vi "Main.vi"(11 "Module Admin":refnum<class "Delacor_lib_QMH_Module Admin.lvclass">) -> ()   [LabVIEW 2020, in "Panther Dashboard.lvlib"]
doc: "Panther Dashboard For DQMH®\n\nDeveloped and maintained by:\nPantherLAB\n\nDeveloper:\n\n» Enrique Noé Arias"
uses:
  Panther Dashboard.lvlib
  <vilib>/Delacor/Delacor QMH/Libraries/Module Admin_class/Delacor_lib_QMH_Module Admin.lvclass
  Controls/Add Event.ctl
  Controls/Remove Event.ctl
  Controls/Convert Event.ctl
  Controls/Rename event.ctl
  Controls/Info.ctl
  Controls/Add New Module.ctl
  Controls/Rename Module.ctl
  Controls/Validate Module.ctl
  Controls/Template.ctl
  Controls/Unit Test.ctl
  Controls/Create Real Time API.ctl
  Controls/Antidoc Open.ctl
  Controls/Antidoc Create.ctl
  Controls/DQMH Help.ctl
  Controls/Add Helper Loop.ctl
  Controls/home.ctl
  Controls/Duplicate Event.ctl
  Controls/Duplicate Module.ctl
  Controls/Configuration.ctl
  Controls/Call HSE-Ify.ctl
  Module Data--cluster.ctl
  Class/Project/Project.lvclass
  C:/GitClones/PantherDashboard/src/LabVIEW/Panther Dashboard/Class/LabVIEWItem/LabVIEWItem.lvclass
  Class/Library/Library.lvclass
  Class/VI/VI.lvclass
  Class/LabVIEWItem/Item Type--enum.ctl
  Module type--enum.ctl
  DQMH Tools Menu--enum.ctl
  Launch DQMH Scripting Tools Argument--cluster.ctl
  <vilib>/Delacor/Delacor QMH/Libraries/Message Queue_class/Delacor_lib_QMH_Message Queue.lvclass/Delacor_lib_QMH_Message Queue.ctl
  Execute Default Event Request Argument--cluster.ctl
  Tree DQMH Selection Argument--cluster.ctl
  Scan DQMH Modules Argument--cluster.ctl
  Stop Argument--cluster.ctl
  Generate Project Documentation Argument--cluster.ctl
  Show About Argument--cluster.ctl
  Update Module ID Argument--cluster.ctl
  Save Library Description Argument--cluster.ctl
  Save VI Description Argument--cluster.ctl
  Open Documentation Argument--cluster.ctl
  Save Project Documentation Argument--cluster.ctl
  Load Project From Path Argument--cluster.ctl
  Add DQMH Module to Current Scan Argument--cluster.ctl
  Highlight Item Argument--cluster.ctl
  Add new Module by Path Argument--cluster.ctl
  Refresh Module By Name Argument--cluster.ctl
  Remove Module By Name Argument--cluster.ctl
  <vilib>/Delacor/Delacor QMH/Libraries/Module Admin_class/Delacor_lib_QMH_Module Admin.lvclass/Delacor_lib_QMH_Module Admin.ctl
  Class/Project/Project.lvclass/Project.ctl
  Public VIs names--enum.ctl
  Class/LabVIEWItem/LabVIEWItem.lvclass/LabVIEWItem.ctl
  Documentation--cluster.ctl
  Class/Library/Library.lvclass/Library.ctl
  <vilib>/Delacor/Delacor QMH/Libraries/Message Queue_class/Delacor_lib_QMH_Enqueue Message (Single).vi
  <vilib>/Delacor/Delacor QMH/Libraries/Module Admin_class/Delacor_lib_QMH_Get External Launch.vi
  Class/LabVIEWItem/Read Item Name.vi
  Class/LabVIEWItem/Read Item Path.vi
  Class/LabVIEWItem/Read Item Type.vi
  Class/Project/Read Project Ref.vi
  Class/LabVIEWItem/Read Item Description.vi
  Class/Library/Read Type.vi
  Class/LabVIEWItem/Write Item Description.vi
  Panther Dashboard--global.vi
  <vilib>/Platform/browser.llb/Open URL in Default Browser (path).vi
  <vilib>/Utility/error.llb/Error Cluster From Error Code.vi
  <vilib>/ErrorRing/Error Ring.xnode
  <vilib>/Delacor/Delacor QMH/Libraries/Message Queue_class/Delacor_lib_QMH_Message Queue.lvclass
  <vilib>/Delacor/Delacor QMH/Libraries/Scripting API/DQMH_Scripting API.lvlib
  ContextHelp/ContextHelp.lvlib
  Class/LabVIEWItem/LabVIEWItem.lvclass
panel:
  in  "Context Help Panther":T1 caption="Doc Editor"
  in  "Duplicate Event":T2
  in  "Add Event":T3
  in  "Remove Event":T4 caption="Remove"
  in  "Convert Event":T5 caption="Convert"
  in  "Rename Event":T6 caption="Rename"
  in  "HSE-Ifi Module":T7
  in  "Duplicate Module":T8
  in  "Add Helper Loop to Module":T9
  in  "Add New Module":T10 caption="Add"
  in  "Rename Module":T11 caption="Rename"
  in  "Validate Module":T12 caption="Validate"
  in  "Create Module Template":T13 caption="Template"
  in  "Add Unit Test Module":T14 caption="Unit Test"
  in  "Create RT Tester Module":T15 caption="RT Tester"
  in  "Open Antidoc Output":T16 caption="Open"
  in  "Generate Antidoc":T17 caption="Antidoc"
  in  "Config":T18
  in  "About Panther":T19 caption="About"
  in  "Home":T20
  in  "Modules Tree":string(tree)
  in  "Module ID":i32=-1 min=-1 max=1000 step=1 format="Module ID %d"
  out "String Control":string
  out "error out":errorcluster
  out "Progress":i16(slide) scale=-1.0..11.0
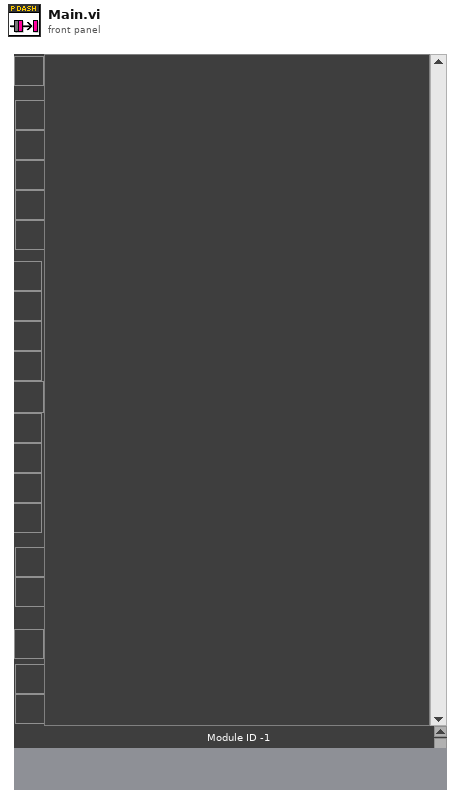
[diagram p1: front panel]
types:
  T1 = typedef "DQMH Help.ctl" = bool
  T2 = typedef "Duplicate Event.ctl" = bool
  T3 = typedef "Add Event.ctl" = bool
  T4 = typedef "Remove Event.ctl" = bool
  T5 = typedef "Convert Event.ctl" = bool
  T6 = typedef "Rename event.ctl" = bool
  T7 = typedef "Call HSE-Ify.ctl" = bool
  T8 = typedef "Duplicate Module.ctl" = bool
  T9 = typedef "Add Helper Loop.ctl" = bool
  T10 = typedef "Add New Module.ctl" = bool
  T11 = typedef "Rename Module.ctl" = bool
  T12 = typedef "Validate Module.ctl" = bool
  T13 = typedef "Template.ctl" = bool
  T14 = typedef "Unit Test.ctl" = bool
  T15 = typedef "Create Real Time API.ctl" = bool
  T16 = typedef "Antidoc Open.ctl" = bool
  T17 = typedef "Antidoc Create.ctl" = bool
  T18 = typedef "Configuration.ctl" = bool
  T19 = typedef "Info.ctl" = bool
  T20 = typedef "home.ctl" = bool
  T21 = typedef "Panther Dashboard.lvlib/Broadcast Events--cluster.ctl" = cluster{"Module Did Init":refnum<user-event>, "Status Updated":refnum<user-event>, "Error Reported":refnum<user-event>, "Module Did Stop":refnum<user-event>, "Update Module Execution Status":refnum<user-event>, "References Updated":refnum<user-event>, "Progress updated":refnum<user-event>, "Scale Updated":refnum<user-event>, "Connector Pane Updated":refnum<user-event>, "Documentation Updated":refnum<user-event>, "Module Type Updated":refnum<user-event>, "Project Description Updated":refnum<user-event>}
  T22 = typedef "Panther Dashboard.lvlib/Request Events--cluster.ctl" = cluster{"Stop Module":refnum<user-event>, "Show Panel":refnum<user-event>, "Hide Panel":refnum<user-event>, "Get Module Execution Status":refnum<user-event>, "Show Diagram":refnum<user-event>, "Scan DQMH Modules":refnum<user-event>, "Tree DQMH Selection":refnum<user-event>, "Open Module API Tester":refnum<user-event>, "Execute Default Event Request":refnum<user-event>, "Launch DQMH Scripting Tools":refnum<user-event>, "Generate Project Documentation":refnum<user-event>, "Show About":refnum<user-event>, "Update Module ID":refnum<user-event>, "Save Library Description":refnum<user-event>, "Save VI Description":refnum<user-event>, "Open Documentation":refnum<user-event>, "Save Project Documentation":refnum<user-event>, "Register controls Mouse Enter":refnum<user-event>, "Load Project From Path":refnum<user-event>, "Add DQMH Module to Current Scan":refnum<user-event>, "Highlight Item":refnum<user-event>, "Update Status":refnum<user-event>, "Add new Module by Path":refnum<user-event>, "Refresh Module By Name":refnum<user-event>, "Remove Module By Name":refnum<user-event>}
  T23 = typedef "ContextHelp.lvlib/Broadcast Events--cluster.ctl" = cluster{"Module Did Init":refnum<user-event>, "Status Updated":refnum<user-event>, "Error Reported":refnum<user-event>, "Module Did Stop":refnum<user-event>, "Update Module Execution Status":refnum<user-event>}
  T24 = typedef "Panther Dashboard.lvlib/LabVIEWItem.lvclass/Item Type--enum.ctl" = enum16{"Requests", "Broadcasts", "Request and Wait for Reply", "Round Trip", "» Public API VIs", "» Constant VIs", "» Error VIs", "Module", "Project", "No Drag Selection"}
  T25 = typedef "Panther Dashboard.lvlib/Module Data--cluster.ctl" = cluster{"Project":refnum<class "Project.lvclass">, "Current Selection":cluster{"Library":refnum<class "Library.lvclass">, "VI":refnum<class "VI.lvclass">}, "Module ID":i32, "Tree Selection":string}
  T26 = typedef "Panther Dashboard.lvlib/Module type--enum.ctl" = enum16{"Singleton", "Cloneable"}
  T27 = typedef "Panther Dashboard.lvlib/Launch DQMH Scripting Tools Argument--cluster.ctl" = cluster{"Scripting Tool":T28}
  T28 = typedef "Panther Dashboard.lvlib/DQMH Tools Menu--enum.ctl" = enum16{"Create New DQMH Event", "Remove DQMH Event", "Convert DQMH Event", "Rename DQMH Event", "Add New DQMH Module", "Create RT Tester", "Rename DQMH Module", "Validate DQMH Module", "Create DQMH Module Template", "New DQMH  Unit Test", "Add Helper Loop to DQMH Module", "Duplicate Event", "HSE-ify DQMH Module", "Duplicate Module"}
  T29 = typedef "Panther Dashboard.lvlib/Execute Default Event Request Argument--cluster.ctl" = cluster{"Event Name":string}
  T30 = typedef "Panther Dashboard.lvlib/Tree DQMH Selection Argument--cluster.ctl" = cluster{"Tree Sel":string}
  T31 = typedef "Panther Dashboard.lvlib/Scan DQMH Modules Argument--cluster.ctl" = cluster{"Include Dependencies":bool, "Scan All":bool, "Project":string, "Target":string}
  T32 = enum32{"invalid lock state", "Not Locked", "Locked (No Password)", "Password-protected"}
  T33 = typedef "Panther Dashboard.lvlib/Stop Argument--cluster.ctl" = cluster{"Origin":string, "Exit via Stop Module Req?":bool, "Wait for Module to stop?":bool}
  T34 = typedef "Panther Dashboard.lvlib/Generate Project Documentation Argument--cluster.ctl" = cluster{"Boolean":bool}
  T35 = typedef "Panther Dashboard.lvlib/Show About Argument--cluster.ctl" = cluster{"Boolean":bool}
  T36 = typedef "Panther Dashboard.lvlib/Update Module ID Argument--cluster.ctl" = cluster{"New ID":i32}
  T37 = typedef "Panther Dashboard.lvlib/Save Library Description Argument--cluster.ctl" = cluster{"Library Description":string}
  T38 = typedef "Panther Dashboard.lvlib/Save VI Description Argument--cluster.ctl" = cluster{"VI Description":string}
  T39 = typedef "Panther Dashboard.lvlib/Open Documentation Argument--cluster.ctl" = cluster{"Boolean":bool}
  T40 = typedef "Panther Dashboard.lvlib/Save Project Documentation Argument--cluster.ctl" = cluster{"Project Description":string}
  T41 = typedef "Panther Dashboard.lvlib/Load Project From Path Argument--cluster.ctl" = cluster{"Project Path":path}
  T42 = typedef "Panther Dashboard.lvlib/Add DQMH Module to Current Scan Argument--cluster.ctl" = cluster{"Include Dependencies":bool}
  T43 = typedef "Panther Dashboard.lvlib/Highlight Item Argument--cluster.ctl" = cluster{"Item Tag":string}
  T44 = typedef "Panther Dashboard.lvlib/Add new Module by Path Argument--cluster.ctl" = cluster{"Module Folder":path, "Module Name":string}
  T45 = typedef "Panther Dashboard.lvlib/Refresh Module By Name Argument--cluster.ctl" = cluster{"Module Name":string}
  T46 = typedef "Panther Dashboard.lvlib/Remove Module By Name Argument--cluster.ctl" = cluster{"Module Name":string}
  T47 = typedef "Panther Dashboard.lvlib/Public VIs names--enum.ctl" = enum16{"Start Module.vi", "Synchronize Module Events.vi", "Obtain Broadcast Events for Registration.vi", "Null Broadcast Events--constant.vi", "Stop Module.vi", "Load Module.vi", "Obtain Default Broadcast Events.vi"}
  T48 = typedef "Panther Dashboard.lvlib/Documentation--cluster.ctl" = cluster{"Module Description":string, "Event Description":string}
  T49 = typedef "Panther Dashboard.lvlib/Pdash Style--cluster.ctl" = cluster{"Gris Obscuro Azul":u32, "Gris Medio Azul":u32, "Gris Claro Azul":u32, "Amarillo":u32, "Text color":u32, "Transparent":u32, "Fuente":string, "Text.Font:Size":u32}
  T50 = cluster{"Library":refnum<class "Library.lvclass">, "VI":refnum<class "VI.lvclass">}
  T51 = typedef "Panther Dashboard.lvlib/Helper Loop--cluster.ctl" = cluster{"Main.vi Refs":refnum<vi>[], "Libraries Names":string[], "Modules Types":T26[], "Dependencies":bool[], "Project Name":string, "HSE Module":bool[], "Glyphs Map":map{T52, i32}, "TreeControl Ref":refnum<vi>}
  T52 = typedef "Panther Dashboard.lvlib/Glyphs--enum.ctl" = enum16{"Singleton", "SingletonRun", "SingletonDepencencies", "SingletonDependenciesRun", "Cloneable", "CloneableRun", "CloneableDependencies", "CloneableDependenciesRun", "HSE_Singleton", "HSE_SingletonRun", "HSE_SingletonDependencies", "HSE_SingletonDependenciesRun", "HSE_Cloneable", "HSE_CloneableRun", "HSE_CloneableDependencies", "HSE_CloneableDependenciesRun", "DQMH_Proj", "HSE_Proj", "Bad"}
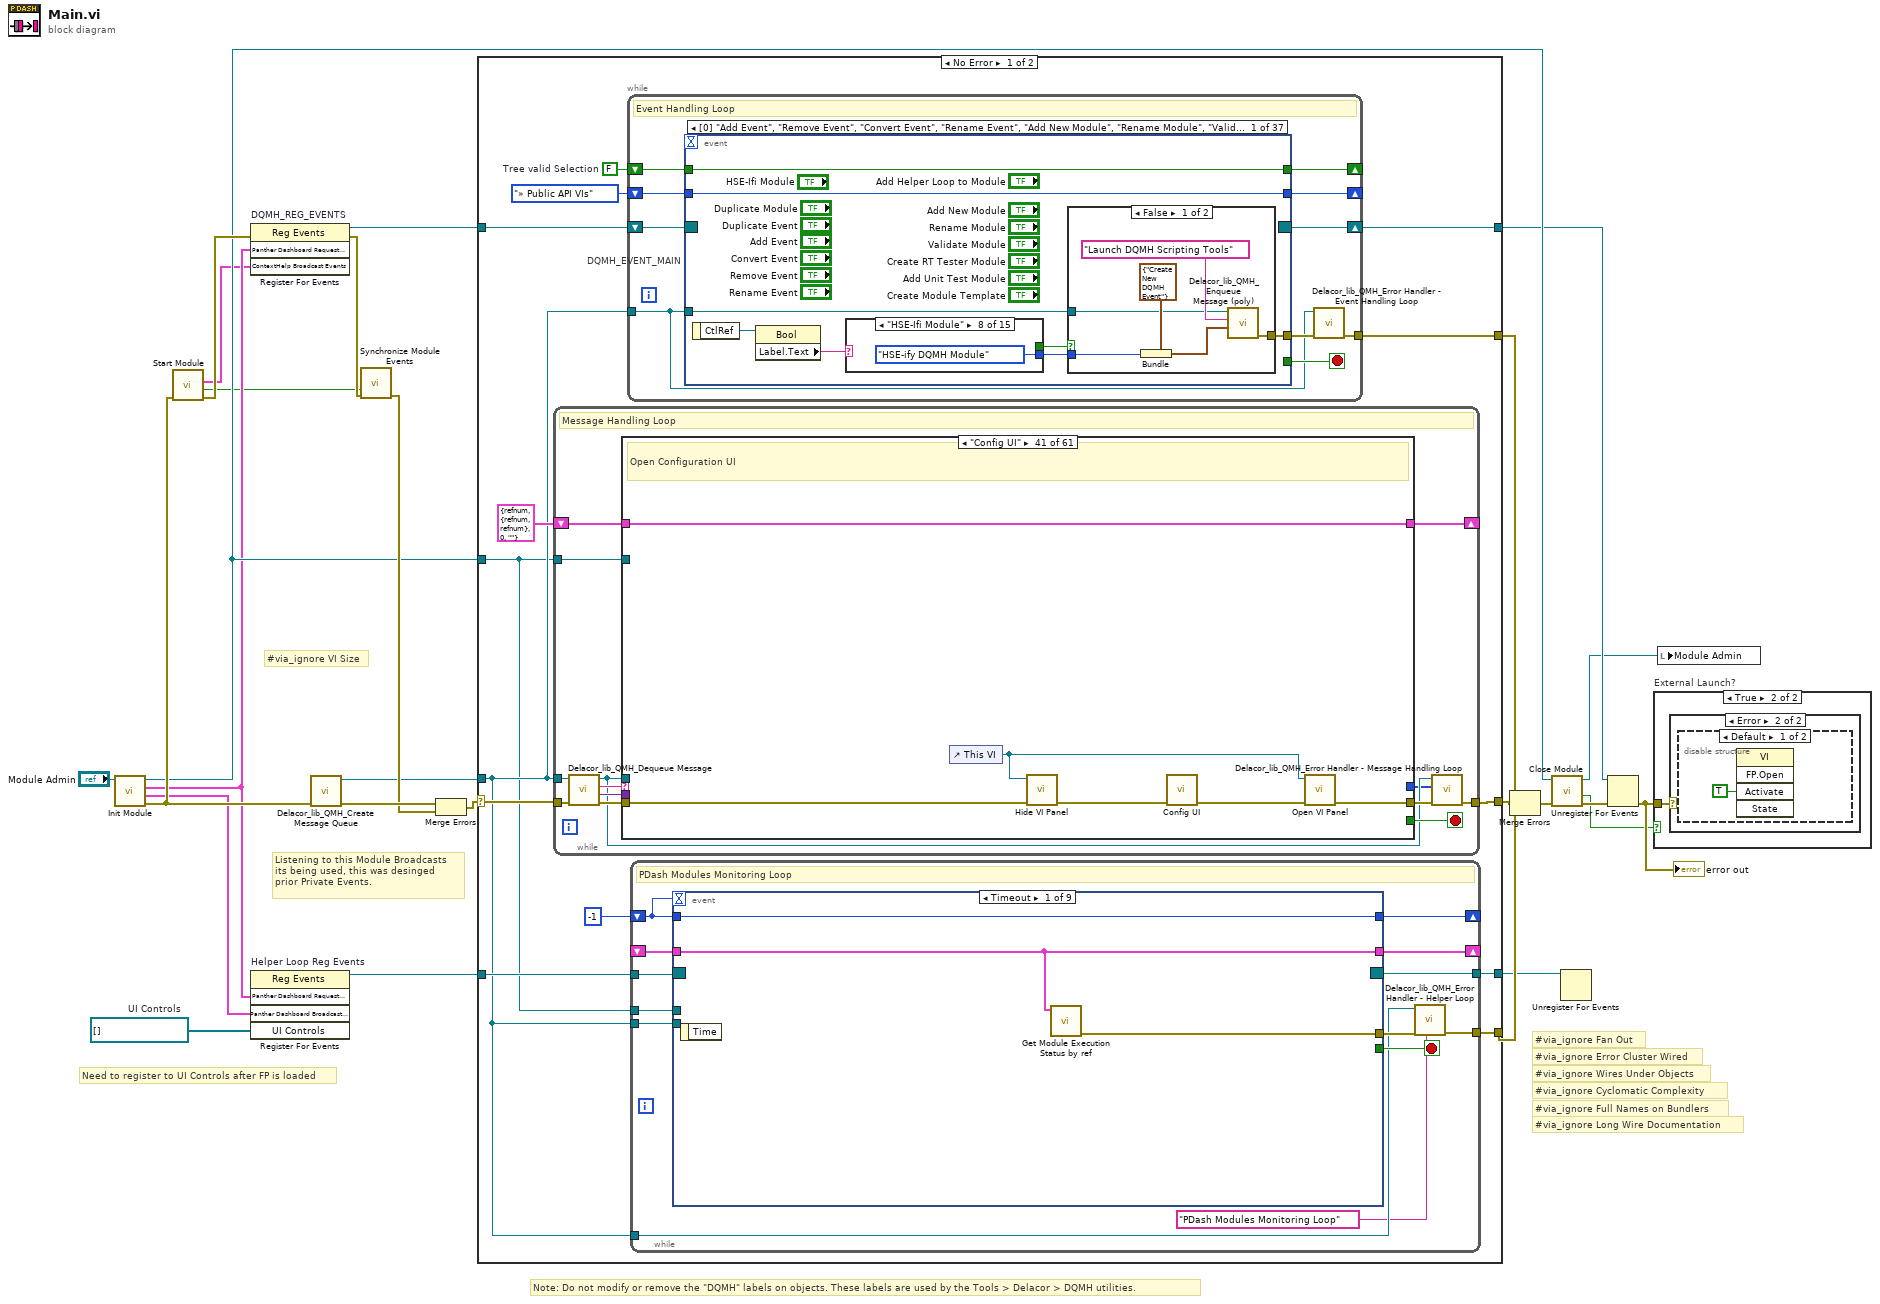
[diagram p0: block diagram]
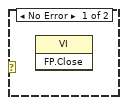
[diagram p3: hidden frame]
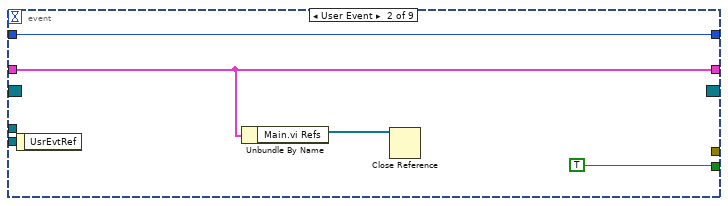
[diagram p5: hidden frame]
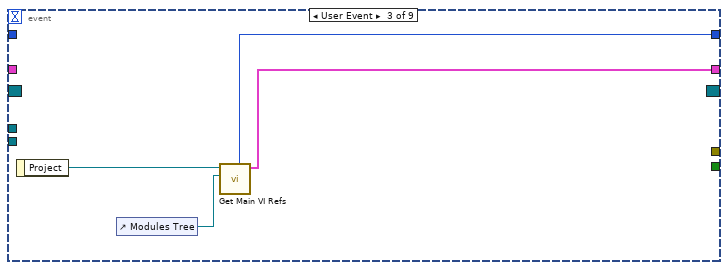
[diagram p6: hidden frame]
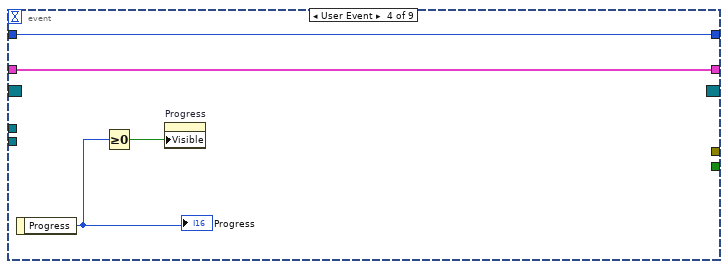
[diagram p7: hidden frame]
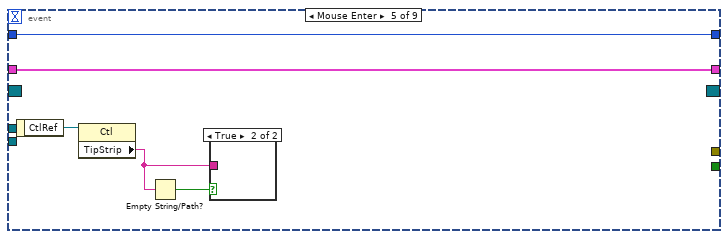
[diagram p8: hidden frame]
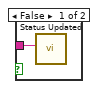
[diagram p9: hidden frame]
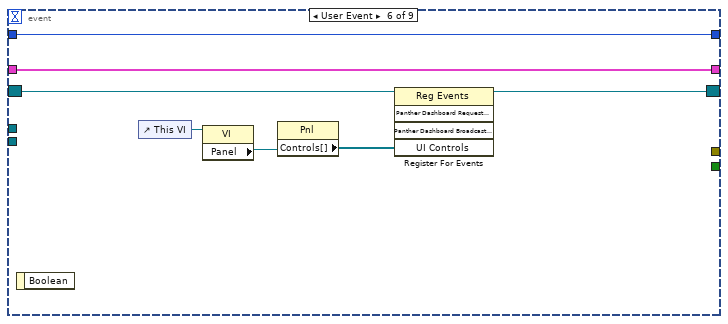
[diagram p10: hidden frame]
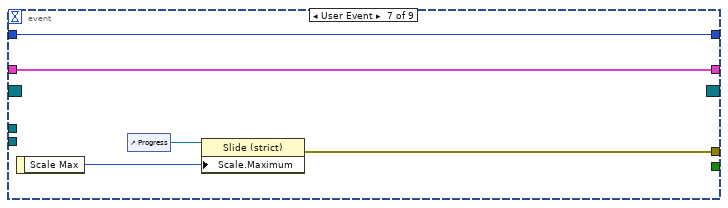
[diagram p11: hidden frame]
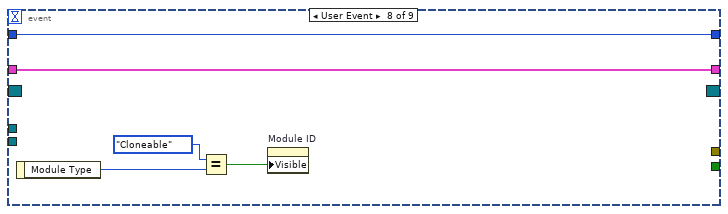
[diagram p12: hidden frame]
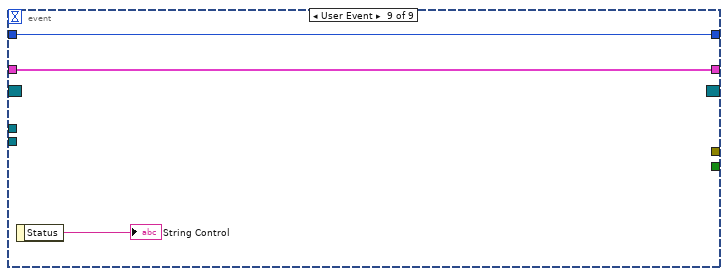
[diagram p13: hidden frame]
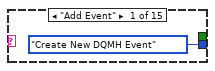
[diagram p15: hidden frame]
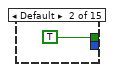
[diagram p16: hidden frame]
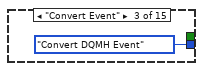
[diagram p17: hidden frame]
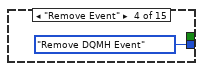
[diagram p18: hidden frame]
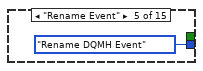
[diagram p19: hidden frame]
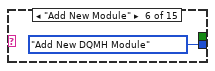
[diagram p20: hidden frame]
diagram:
  w1 = refnum<vi>[] []  # UI Controls
  # "Listening to this Module Broadcasts\nits being used, this was desinged\nprior Private Events."
  # "#via_ignore Long Wire Documentation"
  # "#via_ignore Full Names on Bundlers"
  # "Need to register to UI Controls after FP is loaded"
  # "#via_ignore VI Size"
  # "#via_ignore Fan Out"
  # "#via_ignore Cyclomatic Complexity"
  # "#via_ignore Wires Under Objects"
  # "#via_ignore Error Cluster Wired"
  # "Note: Do not modify or remove the \"DQMH\" labels on objects. These labels are used by the Tools > Delacor > DQMH utilities."
  n1 = call "Init Module.vi"("Singleton Module Admin in"="Module Admin") -> ("error out"=w15:errorcluster, "Panther Dashboard Broadcast Events"=w4:T21, "Panther Dashboard Request Events"=w5:T22, "Singleton Module Admin out"=w14:refnum<class "Delacor_lib_QMH_Module Admin.lvclass">)  [unwired: 7 in]
  n2 = call "Start Module.vi"("error in"=w15) -> ("error out"=w17:errorcluster, "Wait for Event Sync?"=w3:bool, "ContextHelp Broadcast Events"=w2:T23)  [unwired: 6 in, 2 out]
  n3 = register-events "DQMH_REG_EVENTS"(error in=w17, w5, w2) -> (reference out=w12:refnum<event-registration>, error out=w18:errorcluster)  [unwired: 1 in]
  n4 = register-events "Helper Loop Reg Events"(w5, w4, w1) -> (reference out=w7:refnum<event-registration>)  [unwired: 2 in, 1 out]
  n5 = call <vilib>:"Delacor_lib_QMH_Create Message Queue.vi"("error in"=w15) -> ("error out"=w21:errorcluster, "Message Queue"=w11:refnum<class "Delacor_lib_QMH_Message Queue.lvclass">)  [unwired: 9 in]
  n6 = call "Synchronize Module Events.vi"("error in"=w18, "Wait for Event Sync?"=w3) -> ("error out"=w16:errorcluster)  [unwired: 9 in]
  n7 = Merge Errors(w21, w16) -> (w20:errorcluster)
  n8 = case shown="No Error" w20 {
    selector: w20 -> [w38 w1095]
    tunnel: [w40 w1094] -> w26
    tunnel: [w36 w1093] -> w13
    tunnel: w12 -> [w34 w1093]
    tunnel: w11 -> [w29 w1089]
    tunnel: [w39 _] -> w24
    tunnel: w14 -> [w28 w1090]
    tunnel: w7 -> [w33 w1088]
    tunnel: [w32 w1088] -> w6
    tunnel: [w37 _] -> w19
    frame No Error {
      w30 = FALSE  # Tree valid Selection
      n9 = while {
        tunnel: w29 -> [w456]
        shift-right: [w460] -> _
        shift-left: T25 {"Project"=refnum, "Current Selection"={"Library"=refnum, "VI"=refnum}, "Module ID"=0, "Tree Selection"=""} ("Data Cluster") -> [w461]
        tunnel: w38 -> [w464]
        tunnel: [w462] -> w40
        tunnel: w28 -> [w454]
        stop <- w459 stop-if-true
        # "Message Handling Loop"
        n10 = call-dynamic "Delacor_lib_QMH_Dequeue Message.vi"("error in"=w464, "Message Queue in"=w456) -> ("error out"=w463:errorcluster, "Message Data"=w457:variant, "Message"=w458:string, "Message Queue out"=w455:refnum<class "Delacor_lib_QMH_Message Queue.lvclass">)  [unwired: 6 in]
        n11 = case "DQMH_MESSAGE_CASES" shown="\"Config UI\"" w458 {
          selector: w458 -> [_ _ _ _ _ _ _ _ _ _ _ _ _ _ _ _ _ _ _ _ _ _ _ _ _ _ _ _ _ _ _ _ _ _ _ _ _ _ _ _ _ _ _ _ _ _ _ _ _ _ _ _ _ _ _ _ _ w1037 _ _ _]
          tunnel: w455 -> [_ _ _ _ _ _ _ _ _ _ _ _ _ _ _ _ w606 w629 _ _ _ _ _ _ _ _ _ _ _ _ _ _ _ _ _ _ _ _ _ _ _ _ _ _ w871 _ _ _ _ _ _ _ _ _ _ w1002 w1029 _ _ _ _]
          tunnel: w463 -> [w485 w488 w494 w501 w507 w515 w526 w540 w545 w548 w561 w570 w575 w581 w586 w594 w608 w631 w648 w654 w663 w668 w670 w678 w680 w689 w694 w707 w726 w754 _ w766 w774 w777 w794 w809 w814 w819 w821 w830 w836 w844 w866 w868 w882 w892 w898 w909 w912 w921 w931 w951 w974 w988 w999 w1009 w1035 w1039 w1059 w1076 w1086]
          tunnel: [w483 w488 w495 w502 w509 w514 w525 w538 w544 w549 w558 w568 w573 w579 w587 w595 w607 w630 w647 w653 w662 w667 w670 w675 w680 w685 w693 w705 w724 w755 w763 w767 w772 w787 w793 w803 w813 w818 w821 w826 w833 w843 w865 w868 w881 w891 w896 w910 w912 w919 w928 w949 w970 w986 w999 w1005 w1032 w1040 w1057 w1074 w1085] -> w465
          tunnel: w461 -> [w475 w487 w492 w499 w506 w513 w517 w531 w542 w547 w557 w567 w572 w578 w585 w593 w602 w624 w646 w652 w661 w666 w669 w674 w679 w684 w692 w700 w723 w752 w760 w765 w771 w783 w792 w802 w812 w817 w820 w825 w832 w842 w858 w867 w875 w890 w895 w905 w911 w915 w924 w943 w962 w981 w998 w1004 w1019 w1038 w1053 w1069 w1080]
          tunnel: [w481 w487 w492 w499 w506 w513 w520 w528 w541 w546 w556 w567 w572 w578 w585 w593 w600 w623 w646 w652 w661 w666 w669 w674 w679 w684 w692 w700 w723 w752 w760 w765 w771 w783 w790 w802 w812 w817 w820 w825 w832 w838 w850 w867 w874 w890 w895 w905 w911 w915 w922 w942 w962 w980 w998 w1004 w1019 w1038 w1052 w1068 w1079] -> w460
          tunnel: [_ _ _ _ _ _ _ _ _ _ _ _ _ _ _ _ _ _ _ _ _ _ _ _ _ _ _ _ _ _ _ _ _ _ _ _ _ _ _ _ _ _ _ _ _ _ _ _ _ _ _ _ _ _ _ _ w1028 _ _ _ _] -> w459
          tunnel: w457 -> [_ _ _ _ _ _ w522 w537 _ _ _ w566 _ _ _ _ _ _ _ _ _ _ _ _ _ _ _ w703 _ _ _ _ _ _ w791 _ _ _ _ w824 _ w841 w861 _ w878 _ _ _ _ w917 w927 w947 w969 w985 _ w1003 w1027 _ w1056 w1073 w1083]
          tunnel: w454 -> [w482 _ _ _ _ _ _ _ _ _ _ _ _ _ _ _ _ _ _ _ _ _ _ _ _ _ _ _ _ _ _ _ _ _ _ _ _ _ _ _ _ _ _ _ _ _ _ _ _ _ _ _ _ _ _ w1001 w1022 _ _ _ _]
          tunnel: [_ _ _ _ _ _ _ _ _ _ _ _ _ _ _ _ _ _ _ _ _ _ _ _ _ _ _ _ i32[] [5000, 1026, 43] ("specific error code to clear (0: all)") _ _ _ _ _ _ _ _ _ _ _ _ _ _ _ _ _ _ _ _ _ _ _ _ _ _ _ _ _ _ _ _] -> w453
          frame "Initialize" {
            # "Initialize - Any operation that needs to be done before the module can receive messages. Synchronize Caller Events.vi will inform Start Module.vi that the module has launched and is ready to receive messages. Module Did Init.vi will broadcast that the module initialized."
            n12 = call "Synchronize Caller Events.vi"("error in (no error)"=w485, "Singleton Module Admin in"=w482) -> ("error out"=w484:errorcluster, "Singleton Module Admin out"=w474:refnum<class "Delacor_lib_QMH_Module Admin.lvclass">)  [unwired: 8 in]
            n13 = property on="Modules Tree" class="Tree (strict)"("Allow Item Drag"=TRUE ("Drag/Drop:Allow Dragging"), "SelColor"=u32 5987163) -> ()  [unwired: 2 in, 2 out]
            n14 = call "Module Name--constant.vi"() -> ("Module Name"=w479:string)  [unwired: 11 in]
            n15 = call "Module Did Init.vi"("error in (no error)"=w484, "Initialized?"=TRUE, "Origin"=w479) -> ("error out"=w483:errorcluster)  [unwired: 8 in]
            n16 = property class="Module Admin"(reference=w474) -> ("Accessors:External Launch"=w473:bool)  [unwired: 1 in, 2 out]
            n17 = case shown="False" w473 {
              frame False {
                n18 = call "Show Panel.vi"() -> ()  [unwired: 11 in, 1 out]
              }
              frame True {
              }
            }
            n19 = call "Get Panther Dashboard Version.vi"() -> ("Panther Dashboard Version"=w470:string)  [unwired: 11 in]
            n20 = Format Into String(format string="Panther Dashboard for DQMH %s" ("String"), w470) -> (resulting string=w469:string)  [unwired: 2 in, 1 out]
            n21 = control-ref of="This VI"() -> (w472:refnum<vi>)
            n22 = flat-sequence {
              tunnel: [w486] -> w468
              frame #0 {
                n23 = call "PDash Branding.vi"() -> ()  [unwired: 12 in]
                n24 = call "Pdash Style--constant.vi"() -> ("Style"=w486:T49)  [unwired: 11 in]
              }
            }
            n25 = property class="VI"(reference=w472, "Front Panel.Title"=w469) -> ()  [unwired: 1 in, 2 out]
            n26 = Unbundle By Name(w468) -> ("Gris Medio Azul"=w467:u32)
            n27 = call "Status Updated.vi"("Status"=w469) -> ()  [unwired: 10 in, 1 out]
            n28 = control-ref of="Pane Bottom"() -> (w466:refnum<vi>)
            n29 = Bundle By Name(cluster=w475, "Module ID"=-1) -> (w481:T25)
            n30 = property class="Pane"(reference=w466, "PaneColor"=w467) -> ()  [unwired: 1 in, 2 out]
          }
          frame "--------MODULE-----------" {
          }
          frame "Module Data--cluster.ctl" {
            # "Open Module's Data Typedef"
            n31 = Unbundle By Name(w492) -> ("Project"=w490:refnum<class "Project.lvclass">, "Current Selection.Library"=w491:refnum<class "Library.lvclass">)
            n32 = call "Read Main App Inst Ref.vi"("error in (no error)"=w494, "Project in"=w490) -> ("error out"=w493:errorcluster, "Main App Inst Ref"=w489:refnum<vi>)  [unwired: 7 in, 1 out]
            n33 = call "Open Module Data Typedef.vi"("App Instance"=w489, "error in"=w493, "Library in"=w491) -> ("error out"=w495:errorcluster)  [unwired: 7 in, 1 out]
          }
          frame "Main.vi Block Diagram" {
            n34 = Unbundle By Name(w499) -> ("Project"=w497:refnum<class "Project.lvclass">, "Current Selection.Library"=w498:refnum<class "Library.lvclass">)
            n35 = call "Read Main App Inst Ref.vi"("error in (no error)"=w501, "Project in"=w497) -> ("error out"=w500:errorcluster, "Main App Inst Ref"=w496:refnum<vi>)  [unwired: 7 in, 1 out]
            n36 = call "Open Module Main Block Diagram.vi"("App Instance"=w496, "error in"=w500, "Library in"=w498) -> ("error out"=w502:errorcluster)  [unwired: 7 in, 1 out]
          }
          frame "Main.vi Front Panel" {
            n37 = Unbundle By Name(w506) -> ("Project"=w504:refnum<class "Project.lvclass">, "Current Selection.Library"=w505:refnum<class "Library.lvclass">)
            n38 = call "Read Main App Inst Ref.vi"("error in (no error)"=w507, "Project in"=w504) -> ("error out"=w508:errorcluster, "Main App Inst Ref"=w503:refnum<vi>)  [unwired: 7 in, 1 out]
            n39 = call "Open Module Main Front Panel.vi"("App Instance"=w503, "error in"=w508, "Library in"=w505) -> ("error out"=w509:errorcluster)  [unwired: 7 in, 1 out]
          }
          frame "API Tester" {
            w510 = TRUE  # Run API Tester?
            # "Open the API Tester from the current DQMH Module Selected"
            n40 = Unbundle By Name(w513) -> ("Project"=w511:refnum<class "Project.lvclass">, "Current Selection.Library"=w512:refnum<class "Library.lvclass">)
            n41 = call "Open API Tester.vi"("Run API Tester?"=w510, "error in"=w515, "Library"=w512, "Project"=w511) -> ("error out"=w514:errorcluster)  [unwired: 7 in]
          }
          frame "Scan DQMH Modules" {
            # "Scan DQMH Modules in the project, builds a Project Object and draws a Tree with the scanned Project."
            n42 = Variant To Data(error in=w526, type=T31 {"Include Dependencies"=FALSE, "Scan All"=FALSE, "Project"="", "Target"=""} ("Scan DQMH Modules Argument"), Variant=w522) -> (data=w518:T31, error out=w524:errorcluster)
            n43 = call <vilib>:"Set Busy.vi"("error in (no error)"=w524) -> ()  [unwired: 9 in, 2 out]
            n44 = control-ref of="Modules Tree"() -> (w519:refnum<vi>)
            n45 = call "Scan DQMH Modules from Project.vi"("TreeControl in"=w519, "Data Cluster In"=w517, "error in"=w524, "Scan DQMH Modules Argument"=w518) -> ("error out"=w523:errorcluster, "Data Cluster Out"=w520:T25)  [unwired: 6 in]
            n46 = call <vilib>:"Unset Busy.vi"("error in (no error)"=w523) -> ()  [unwired: 10 in, 1 out]
            n47 = call "Progress updated.vi"("error in"=w523, "Progress"=i16 -1) -> ()  [unwired: 9 in, 1 out]
            n48 = call "Show Panel.vi"("error in (no error)"=w523) -> ("error out"=w525:errorcluster)  [unwired: 10 in]
          }
          frame "Launch DQMH Scripting Tools" {
            # "Launch the DQMH Scripting Tools"
            n49 = Variant To Data(error in=w540, type=T27 {"Scripting Tool"=enum."Create New DQMH Event"} ("Launch DQMH Scripting Tools Argument"), Variant=w537) -> (data=w535:T27, error out=w539:errorcluster)
            n50 = Unbundle By Name(w535) -> ("Scripting Tool"=w532:T28)
            n51 = Format Into String(format string="Executing DQMH: %s", w532) -> (resulting string=w534:string)  [unwired: 2 in, 1 out]
            n52 = call "Status Updated.vi"("Status"=w534) -> ()  [unwired: 10 in, 1 out]
            n53 = Unbundle By Name(w531) -> ("Project"=w530:refnum<class "Project.lvclass">, "Current Selection"=w529:T50)
            n54 = call "Launch DQMH Tools by menu.vi"("error in"=w539, "DQMH Tools"=w532, "Current Selection In"=w529, "Project In"=w530) -> ("error out"=w538:errorcluster, "Project Out"=w527:refnum<class "Project.lvclass">)  [unwired: 6 in]
            n55 = Bundle By Name(cluster=w531, "Project"=w527) -> (w528:T25)
          }
          frame "(X) Exclude Module from Scan" {
            # "To Exclude a Module form the current Scan, this is specially usefull when dealing with dependencies that were removed from the project."
            n56 = control-ref of="Modules Tree"() -> (w543:refnum<vi>)
            n57 = call "Remove Module from Project.vi"("TreeControl in"=w543, "error in"=w545, "Data Cluster In"=w542) -> ("error out"=w544:errorcluster, "Data Cluster Out"=w541:T25)  [unwired: 7 in]
          }
          frame "Scan Project for Manually Added Modules" {
            # "Scan Project for Manually Added Modules"
            n58 = in-place {
              in-place-border: [w554] -> w549
              in-place-border: w548 -> [w553]
              n59 = in-place-cluster #1(w547) -> ("Project"=w551:refnum<class "Project.lvclass">)
              n60 = control-ref of="Modules Tree"() -> (w552:refnum<vi>)
              n61 = call "Add Module To Project.vi"("TreeControl in"=w552, "error in"=w553, "Project"=w551) -> ("error out"=w554:errorcluster, "Project Out"=w550:refnum<class "Project.lvclass">)  [unwired: 7 in]
              n62 = in-place-cluster #1("Project"=w550) -> (w546:T25)
            }
          }
          frame "Refresh Module" {
            # "User right click a module and selected Refresh module, this will rescan the Library for events, will redraw the tree with the current module state.\nUse this functionality when working with DQMH and Panther Dashboard wasn't running, this will put the scan up to date"
            n63 = control-ref of="Modules Tree"() -> (w555:refnum<vi>)
            n64 = call <vilib>:"Set Busy.vi"("error in (no error)"=w561) -> ("error out"=w560:errorcluster)  [unwired: 9 in, 1 out]
            n65 = call "Refresh Module.vi"("TreeControl in"=w555, "Data Cluster In"=w557, "error in"=w560) -> ("error out"=w559:errorcluster, "Data Cluster Out"=w556:T25)  [unwired: 7 in]
            n66 = call <vilib>:"Unset Busy.vi"("error in (no error)"=w559) -> ("error out"=w558:errorcluster)  [unwired: 10 in]
          }
          frame "Highlight Item" {
            # "Highligh item in Tree"
            n67 = Variant To Data(error in=w570, type=T43 {"Item Tag"=""} ("Highlight Item Argument"), Variant=w566) -> (data=w564:T43, error out=w569:errorcluster)
            n68 = Unbundle By Name(w564) -> ("Item Tag"=w562:string)
            n69 = control-ref of="Modules Tree"() -> (w563:refnum<vi>)
            n70 = call "Highlight Item in Tree.vi"("error in"=w569, "Tag"=w562, "TreeControl in"=w563) -> ("error out"=w568:errorcluster)  [unwired: 8 in]
          }
          frame "Home Screen" {
            # "User clicked the Home Button."
            n71 = call "Hide Panel.vi"("error in (no error)"=w575) -> ("error out"=w574:errorcluster)  [unwired: 10 in]
            n72 = Unbundle By Name(w572) -> ("Project"=w571:refnum<class "Project.lvclass">)
            n73 = call "Init Screen.vi"("error in"=w574) -> ("error out"=w573:errorcluster)  [unwired: 10 in]
            n74 = invoke on="Modules Tree" class="Tree (strict)" method="Edit Tree Items.Delete"() -> ()  [unwired: 5 in, 5 out]
            n75 = call "Close refs.vi"("Project"=w571) -> ()  [unwired: 10 in, 1 out]
          }
          frame "Find Module in project explorer" {
            # "Open Project Explorer Window and hilite Current Module"
            n76 = Unbundle By Name(w578) -> ("Current Selection.Library"=w577:refnum<class "Library.lvclass">, "Project"=w576:refnum<class "Project.lvclass">)
            n77 = call "Find Module In Project and Open Main.vi"("error in"=w581, "Project"=w576, "Library in"=w577) -> ("error out"=w580:errorcluster)  [unwired: 8 in]
            n78 = call "Show Panel.vi"("error in (no error)"=w580) -> ("error out"=w579:errorcluster)  [unwired: 10 in]
          }
          frame "Where is this module being Launched?" {
            # "Find all the VIS calling the Start Module.vi of the selected module library"
            n79 = call <vilib>:"Set Busy.vi"("error in (no error)"=w586) -> ("error out"=w589:errorcluster)  [unwired: 9 in, 1 out]
            n80 = Unbundle By Name(w585) -> ("Project"=w584:refnum<class "Project.lvclass">, "Current Selection.Library"=w583:refnum<class "Library.lvclass">)
            n81 = call "Find API VI.vi"("error in"=w589, "Framework VI to Find"=Public_VIs_names--enum."Start Module.vi", "Library"=w583, "Project"=w584) -> ("error out"=w588:errorcluster)  [unwired: 7 in]
            n82 = call <vilib>:"Unset Busy.vi"("error in (no error)"=w588) -> ("error out"=w587:errorcluster)  [unwired: 10 in]
          }
          frame "Where is this module being Stopped?" {
            # "Find all the VIS calling the Obtain broadcast events for registration of the selected module library"
            n83 = call <vilib>:"Set Busy.vi"("error in (no error)"=w594) -> ("error out"=w597:errorcluster)  [unwired: 9 in, 1 out]
            n84 = Unbundle By Name(w593) -> ("Project"=w591:refnum<class "Project.lvclass">, "Current Selection.Library"=w590:refnum<class "Library.lvclass">)
            n85 = call "Find API VI.vi"("error in"=w597, "Framework VI to Find"=Public_VIs_names--enum."Stop Module.vi", "Library"=w590, "Project"=w591) -> ("error out"=w596:errorcluster)  [unwired: 7 in]
            n86 = call <vilib>:"Unset Busy.vi"("error in (no error)"=w596) -> ("error out"=w595:errorcluster)  [unwired: 10 in]
          }
          frame "Create Custom --error.vi" {
            # "Create an error vi for the selected library, it opens a dialog to allow developer adding Controls to the error vi to make it more flexible."
            n87 = call <vilib>:"Set Busy.vi"("error in (no error)"=w608) -> ()  [unwired: 9 in, 2 out]
            n88 = Unbundle By Name(w602) -> ("Project"=w603:refnum<class "Project.lvclass">, "Current Selection.Library"=w604:refnum<class "Library.lvclass">)
            n89 = call "Error Code Dialog.vi"("error in"=w608, "Library"=w604, "Project"=w603) -> ("error out"=w609:errorcluster, "Cancel Out"=w605:bool, "Error Name"=w599:string, "Project out"=w601:refnum<class "Project.lvclass">, "Error VI Tag"=w598:string)  [unwired: 4 in]
            n90 = case shown="False" w605 {
              tunnel: w609 -> [w618 w620]
              tunnel: [w616 w620] -> w607
              tunnel: w606 -> [w614 _]
              tunnel: w602 -> [w613 w619]
              tunnel: w601 -> [w612 _]
              tunnel: [w611 w619] -> w600
              tunnel: w599 -> [_ _]
              tunnel: w598 -> [w610 _]
              frame False {
                n91 = call-poly <vilib>:"Delacor_lib_QMH_Enqueue Message (poly).vi"("error in"=w618, "Message"="Refresh Module", "Message Queue in"=w614) -> ("error out"=w617:errorcluster)  [unwired: 7 in, 1 out]
                n92 = Bundle By Name(cluster=w613, "Project"=w612) -> (w611:T25)
                n93 = call "Highlight Item.vi"("error in"=w617, "Item Tag"=w610) -> ("error out"=w616:errorcluster)  [unwired: 9 in]
              }
              frame True {
                # "User Cancel"
              }
            }
            n94 = call <vilib>:"Unset Busy.vi"("error in (no error)"=w607) -> ()  [unwired: 10 in, 1 out]
          }
          frame "Create Custom --constant.vi" {
            # "Creates a Constant vi to the current Library selection, it opens a dialog to add controls to it, the developer can place values to the controls and those controls will be constants connected to the connector pane."
            n95 = call <vilib>:"Set Busy.vi"("error in (no error)"=w631) -> ()  [unwired: 9 in, 2 out]
            n96 = Unbundle By Name(w624) -> ("Project"=w626:refnum<class "Project.lvclass">, "Current Selection.Library"=w625:refnum<class "Library.lvclass">)
            n97 = call "Custom Constant Dialog.vi"("error in"=w631, "Library"=w625, "Project"=w626) -> ("error out"=w632:errorcluster, "Cancel Out"=w627:bool, "New Constant VI name"=w628:string, "Error VI Tag"=w622:string, "Project out"=w621:refnum<class "Project.lvclass">)  [unwired: 4 in]
            n98 = case shown="False" w627 {
              tunnel: w632 -> [w640 w643]
              tunnel: [w639 w643] -> w630
              tunnel: w629 -> [w635 _]
              tunnel: w628 -> [_ _]
              tunnel: w624 -> [w638 w642]
              tunnel: [w637 w642] -> w623
              tunnel: w622 -> [w636 _]
              tunnel: w621 -> [w634 _]
              frame False {
                n99 = call-poly <vilib>:"Delacor_lib_QMH_Enqueue Message (poly).vi"("error in"=w640, "Message"="Refresh Module", "Message Queue in"=w635) -> ("error out"=w641:errorcluster)  [unwired: 7 in, 1 out]
                n100 = Bundle By Name(cluster=w638, "Project"=w634) -> (w637:T25)
                n101 = call "Highlight Item.vi"("error in"=w641, "Item Tag"=w636) -> ("error out"=w639:errorcluster)  [unwired: 9 in]
              }
              frame True {
              }
            }
            n102 = call <vilib>:"Unset Busy.vi"("error in (no error)"=w630) -> ()  [unwired: 10 in, 1 out]
          }
          frame "Edit 'Module Name--constant.vi' value" {
            # "Sometimes we need to update or modify the 'Module Name--constant.vi' value and we need to go to this vi, open it's block diagram and change the constant value, close the vi and save it, this script does exactly that."
            n103 = Unbundle By Name(w646) -> ("Project"=w645:refnum<class "Project.lvclass">, "Current Selection.Library"=w644:refnum<class "Library.lvclass">)
            n104 = call "Script Edit Module Name.vi"("error in"=w648, "Library"=w644, "Project"=w645) -> ("error out"=w647:errorcluster)  [unwired: 8 in]
          }
          frame "Edit 'Module Timeout--constant.vi' value" {
            w649 = FALSE  # Restore to Default
            # "Sometimes we need to update or modify the 'Module Name--constant.vi' value and we need to go to this vi, open it's block diagram and change the constant value, close the vi and save it, this script does exactly that."
            n105 = Unbundle By Name(w652) -> ("Project"=w651:refnum<class "Project.lvclass">, "Current Selection.Library"=w650:refnum<class "Library.lvclass">)
            n106 = call "Script Module Timeout.vi"("Restore to Default"=w649, "error in"=w654, "Library"=w650, "Project"=w651) -> ("error out"=w653:errorcluster)  [unwired: 7 in]
          }
          frame "Restore Timeout to Default (5000ms)" {
            w660 = TRUE  # Restore to Default
            # "Restore Timeout to Default DQMH Framework value (5000ms)"
            n107 = Unbundle By Name(w661) -> ("Project"=w656:refnum<class "Project.lvclass">, "Current Selection.Library"=w655:refnum<class "Library.lvclass">)
            n108 = property class="Library"(reference=w655) -> ("Accessors:Item Name"=w658:string)  [unwired: 1 in, 2 out]
            n109 = call "Script Module Timeout.vi"("Restore to Default"=w660, "error in"=w663, "Library"=w655, "Project"=w656) -> ("error out"=w662:errorcluster)  [unwired: 7 in]
            n110 = Format Into String(format string="Module: [%s] Timeout set to Framework Default Value (5000ms)", w658) -> (resulting string=w659:string)  [unwired: 2 in, 1 out]
            n111 = call "Status Updated.vi"("error in (no error)"=w662, "Status"=w659) -> ()  [unwired: 9 in, 1 out]
          }
          frame "Open File Library on Disk" {
            # "Open current Module Library selection on the file system"
            n112 = Unbundle By Name(w666) -> ("Current Selection.Library"=w665:refnum<class "Library.lvclass">)
            n113 = property class="Library"(reference=w665) -> ("Accessors:Item Path"=w664:path)  [unwired: 1 in, 2 out]
            n114 = call "Open File on Disk.vi"("error in"=w668, "file or directory path"=w664) -> ("error out"=w667:errorcluster)  [unwired: 9 in]
          }
          frame "---------BROADCASTS---------" {
          }
          frame "Find Code registered to this module's broadcasts" {
            # "Find all the VIS calling the Obtain broadcast events for registration of the selected module library"
            n115 = call <vilib>:"Set Busy.vi"("error in (no error)"=w678) -> ("error out"=w677:errorcluster)  [unwired: 9 in, 1 out]
            n116 = Unbundle By Name(w674) -> ("Project"=w672:refnum<class "Project.lvclass">, "Current Selection.Library"=w671:refnum<class "Library.lvclass">)
            n117 = call "Find API VI.vi"("error in"=w677, "Framework VI to Find"=Public_VIs_names--enum."Obtain Broadcast Events for Registration.vi", "Library"=w671, "Project"=w672) -> ("error out"=w676:errorcluster)  [unwired: 7 in]
            n118 = call <vilib>:"Unset Busy.vi"("error in (no error)"=w676) -> ("error out"=w675:errorcluster)  [unwired: 10 in]
          }
          frame "---------REQUEST--------------" {
          }
          frame "Locate Event on Main" {
            # "Find the selected event vi on the owing DQMH Module, if it is a reques we highlight its frame, if it is a broadcast we highlight where the broadcast is being triggered"
            n119 = call <vilib>:"Set Busy.vi"("error in (no error)"=w689) -> ("error out"=w688:errorcluster)  [unwired: 9 in, 1 out]
            n120 = Unbundle By Name(w684) -> ("Project"=w683:refnum<class "Project.lvclass">, "Current Selection.Library"=w682:refnum<class "Library.lvclass">, "Current Selection.VI"=w681:refnum<class "VI.lvclass">)
            n121 = call "Find Event Frame.vi"("error in"=w688, "VI"=w681, "Library"=w682, "Project"=w683) -> ("error out"=w687:errorcluster)  [unwired: 7 in]
            n122 = call <vilib>:"Unset Busy.vi"("error in (no error)"=w687) -> ("error out"=w686:errorcluster)  [unwired: 10 in]
            n123 = call "Show Panel.vi"("error in (no error)"=w686) -> ("error out"=w685:errorcluster)  [unwired: 10 in]
          }
          frame "Drag VI" {
            # "This is the functionality alowing drag and drop the current selection to your code, you can edit DQMH code using panther Dashboard as it was the Project Explorer"
            n124 = call <vilib>:"Set Busy.vi"("error in (no error)"=w694) -> ()  [unwired: 9 in, 2 out]
            n125 = Unbundle By Name(w692) -> ("Project"=w691:refnum<class "Project.lvclass">, "Current Selection.VI"=w690:refnum<class "VI.lvclass">)
            n126 = call "Drop Event into subVI.vi"("VI"=w690, "Project"=w691) -> ("error out"=w695:errorcluster)  [unwired: 9 in]
            n127 = Merge Errors(w695, w694) -> (w693:errorcluster)
            n128 = call <vilib>:"Unset Busy.vi"("error in (no error)"=w693) -> ()  [unwired: 10 in, 1 out]
          }
          frame "Execute Default Event Request" {
            # "Execute Default Event"
            n129 = Variant To Data(error in=w707, type=T29 {"Event Name"=""} ("Execute Default Event Request Argument"), Variant=w703) -> (data=w701:T29, error out=w706:errorcluster)
            n130 = Unbundle By Name(w700) -> ("Project"=w697:refnum<class "Project.lvclass">, "Current Selection.Library"=w696:refnum<class "Library.lvclass">, "Module ID"=w698:i32)
            n131 = Unbundle By Name(w701) -> ("Event Name"=w699:string)
            n132 = call "Execute Default event.vi"("Module ID"=w698, "Event"=w699, "Library"=w696, "Project"=w697) -> ("error out"=w704:errorcluster)  [unwired: 7 in]
            n133 = Merge Errors(w706, w704) -> (w705:errorcluster)
          }
          frame "Search for Event Callers / listeners" {
            # "1026-Invalid Ref\n43 - Operation\n canceled by user\n5000- something\nrandom happening\non DQMH Scripting\nAPI"
            # "Search for this event callers"
            n134 = Unbundle By Name(w723) -> ("Project"=w719:refnum<class "Project.lvclass">, "Current Selection.VI"=w717:refnum<class "VI.lvclass">)
            n135 = property class="VI"(reference=w717) -> ("Accessors:Item Path"=w714:path, "Accessors:Item Type"=w716:T24)  [unwired: 1 in, 2 out]
            n136 = property class="Project"(reference=w719) -> ("Accessors:Project Ref"=w718:refnum<vi>, "Accessors:Main App Inst Ref"=w713:refnum<vi>)  [unwired: 1 in, 2 out]
            n137 = Equal?(x=w716, y=Item_Type--enum."Broadcasts") -> (x = y?=w710:bool)
            n138 = Open VI Reference(application reference (local)=w713, vi path=w714, error in (no error)=w726) -> (vi reference=w709:refnum<vi>, error out=w725:errorcluster)  [unwired: 3 in]
            n139 = case shown="True" w710 {
              tunnel: [w736 w743] -> w724
              tunnel: [w734 w741] -> w711
              tunnel: w718 -> [w733 w740]
              tunnel: w709 -> [w732 w737]
              tunnel: w725 -> [w735 w742]
              frame False {
                # "Requests"
                n140 = call <vilib>:"Get Callers of Request VI in Project.vi"("error in"=w735, "Request VI"=w732, "Project"=w733) -> ("error out"=w736:errorcluster, "Request VI Callers"=w734:refnum<vi>[])  [unwired: 7 in]
              }
              frame True {
                # "Broadcast"
                n141 = Two Button Dialog(message="This is an exhaustive task that can take up to minutes, do you wish to continue?") -> (T button?=w739:bool)  [unwired: 2 in]
                n142 = case shown="True" w739 {
                  tunnel: [w744 w749] -> w743
                  tunnel: [_ w747] -> w741
                  tunnel: w740 -> [_ w746]
                  tunnel: w737 -> [_ w745]
                  tunnel: w742 -> [w744 w748]
                  frame False {
                  }
                  frame True {
                    n143 = call <vilib>:"Get VIs Registered for Broadcast in Project.vi"("error in"=w748, "Broadcast VI"=w745, "Project"=w746) -> ("error out"=w749:errorcluster, "VIs Registered for Broadcast"=w747:refnum<vi>[])  [unwired: 7 in]
                  }
                }
              }
            }
            n144 = Select(t="Searching code registered to broadcast selection" ("Status"), s=w710, f="Searching for Event Callers" ("Status")) -> (s? t:f=w720:string)
            n145 = call "Status Updated.vi"("error in (no error)"=w725, "Status"=w720) -> ("error out"=w727:errorcluster)  [unwired: 9 in]
            n146 = call <vilib>:"Set Busy.vi"("error in (no error)"=w727) -> ()  [unwired: 9 in, 2 out]
            n147 = call <vilib>:"Unset Busy.vi"("error in (no error)"=w724) -> ()  [unwired: 10 in, 1 out]
            n148 = flat-sequence {
              tunnel: w711 -> [w730]
              tunnel: w710 -> [w729]
              tunnel: w709 -> [w728]
              tunnel: [w728] -> w708
              tunnel: w708 -> [w731]
              frame #0 {
                n149 = call "Show Caller Items Dialog.vi"("Event"=w728, "Find Broadcast?"=w729, "Request VI Callers"=w730) -> ()  [unwired: 9 in]
              }
              frame #1 {
                n150 = Close Reference(reference=w731) -> ()  [unwired: 1 in, 1 out]
              }
            }
          }
          frame "Open VI on Disk" {
            # "Open current event selection on the file system"
            n151 = Unbundle By Name(w752) -> ("Current Selection.VI"=w751:refnum<class "VI.lvclass">)
            n152 = property class="VI"(reference=w751, error in=w754) -> (error out=w753:errorcluster, "Accessors:Item Path"=w750:path)  [unwired: 1 out]
            n153 = call "Open File on Disk.vi"("error in"=w753, "file or directory path"=w750) -> ("error out"=w755:errorcluster)  [unwired: 9 in]
          }
          frame "Open Event Arguments" {
            # "Open The event selected DQMH Arguments, also open the Event BD to do edits on it"
            n154 = Unbundle By Name(w760) -> ("Project"=w758:refnum<class "Project.lvclass">, "Current Selection.Library"=w757:refnum<class "Library.lvclass">, "Current Selection.VI"=w759:refnum<class "VI.lvclass">)
            n155 = call "Open API Tester.vi"("Run API Tester?"=FALSE, "Library"=w757, "Project"=w758) -> ("error out"=w762:errorcluster)  [unwired: 8 in]
            n156 = call "Find Event Frame.vi"("error in"=w762, "VI"=w759, "Library"=w757, "Project"=w758) -> ("error out"=w761:errorcluster)  [unwired: 7 in]
            n157 = call "Open Event Arguments.vi"("error in"=w761, "VI"=w759, "Project"=w758) -> ("error out"=w763:errorcluster)  [unwired: 8 in]
          }
          frame "Set Custom Timeout" {
            # "#TODO, Update The VI on the Project OBJ"
            n158 = Unbundle By Name(w765) -> ("Current Selection.VI"=w764:refnum<class "VI.lvclass">)
            n159 = call "Script Request and Wait For Reply Custom Timeout.vi"("error in"=w766, "VI"=w764) -> ("error out"=w767:errorcluster)  [unwired: 9 in]
          }
          frame "Restore to Module's Timeout" {
            # "#TODO Update VI in the current Project"
            n160 = Unbundle By Name(w771) -> ("Current Selection.Library"=w770:refnum<class "Library.lvclass">, "Current Selection.VI"=w769:refnum<class "VI.lvclass">)
            n161 = call "Script Request and Wait For Reply Restore Timeout.vi"("error in"=w774, "VI"=w769, "Library"=w770) -> ("error out"=w773:errorcluster)  [unwired: 8 in]
            n162 = call "Status Updated.vi"("error in (no error)"=w773, "Status"="Event restored to default Module's Timeout") -> ("error out"=w772:errorcluster)  [unwired: 9 in]
          }
          frame "Open Front Panel" {
            # "User Selection 'Open Front Panel'"
            n163 = Unbundle By Name(w783) -> ("Project"=w779:refnum<class "Project.lvclass">, "Current Selection.VI"=w782:refnum<class "VI.lvclass">)
            n164 = property class="Project"(reference=w779, error in=w777) -> (error out=w775:errorcluster, "Accessors:Main App Inst Ref"=w778:refnum<vi>)  [unwired: 1 out]
            n165 = property class="VI"(reference=w782, error in=w777) -> (error out=w786:errorcluster, "Accessors:Item Path"=w781:path)  [unwired: 1 out]
            n166 = Merge Errors(w775, w786) -> (w776:errorcluster)
            n167 = Open VI Reference(application reference (local)=w778, vi path=w781, error in (no error)=w776) -> (vi reference=w780:refnum<vi>, error out=w785:errorcluster)  [unwired: 3 in]
            n168 = call "Open VI Panel.vi"("error in (no error)"=w785, "VI"=w780) -> ("error out"=w784:errorcluster)  [unwired: 9 in]
            n169 = Close Reference(reference=w780, error in (no error)=w784) -> (error out=w787:errorcluster)
          }
          frame "Module ID Update" {
            # "Module ID Control has value change"
            n170 = Variant To Data(error in=w794, type=0 ("Module ID"), Variant=w791) -> (data=w789:i32, error out=w793:errorcluster)
            n171 = Bundle By Name(cluster=w792, "Module ID"=w789) -> (w790:T25)
          }
          frame "Open VI BD" {
            n172 = Unbundle By Name(w802) -> ("Project"=w796:refnum<class "Project.lvclass">, "Current Selection.VI"=w800:refnum<class "VI.lvclass">)
            n173 = property class="VI"(reference=w800, error in=w809) -> (error out=w805:errorcluster, "Accessors:Item Path"=w799:path)  [unwired: 1 out]
            n174 = property class="Project"(reference=w796, error in=w805) -> (error out=w804:errorcluster, "Accessors:Main App Inst Ref"=w795:refnum<vi>)  [unwired: 1 out]
            n175 = Open VI Reference(application reference (local)=w795, vi path=w799, error in (no error)=w804) -> (vi reference=w798:refnum<vi>, error out=w807:errorcluster)  [unwired: 3 in]
            n176 = property on="Property Node" class="VI"(reference=w798, error in=w807, "BDWin.Open"=TRUE ("Block Diagram Window:Open")) -> (reference out=w797:refnum<vi>, error out=w808:errorcluster)
            n177 = Close Reference(reference=w797, error in (no error)=w808) -> (error out=w806:errorcluster)
            n178 = call "Show Panel.vi"("error in (no error)"=w806) -> ("error out"=w803:errorcluster)  [unwired: 10 in]
          }
          frame "Close and Save Opened VIs" {
            w810 = TRUE  # Save?
            # "Close VIs Opened"
            n179 = Unbundle By Name(w812) -> ("Project"=w811:refnum<class "Project.lvclass">)
            n180 = call "Close and Save Opened VIS.vi"("error in"=w814, "Save?"=w810, "Project in"=w811) -> ("error out"=w813:errorcluster)  [unwired: 8 in]
          }
          frame "Close Opened VIs (No Save)" {
            w815 = FALSE  # Save?
            # "Close VIs Opened"
            n181 = Unbundle By Name(w817) -> ("Project"=w816:refnum<class "Project.lvclass">)
            n182 = call "Close and Save Opened VIS.vi"("error in"=w819, "Save?"=w815, "Project in"=w816) -> ("error out"=w818:errorcluster)  [unwired: 8 in]
          }
          frame "-------PANTHER---------" {
          }
          frame "Show About" {
            # "Show About Panther Dashboard Project"
            n183 = Variant To Data(error in=w830, type=T35 {"Boolean"=FALSE} ("Show About Argument"), Variant=w824) -> (error out=w827:errorcluster)  [unwired: 1 out]
            n184 = control-ref of="This VI"() -> (w822:refnum<vi>)
            n185 = call "Hide VI Panel.vi"("error in (no error)"=w827, "VI"=w822) -> ("error out"=w829:errorcluster)  [unwired: 9 in]
            n186 = call "About Panther Dashboard.vi"("error in"=w829) -> ("error out"=w828:errorcluster)  [unwired: 10 in]
            n187 = call "Open VI Panel.vi"("error in (no error)"=w828, "VI"=w822) -> ("error out"=w826:errorcluster)  [unwired: 9 in]
          }
          frame "Config UI" {
            # "Open Configuration UI"
            n188 = control-ref of="This VI"() -> (w831:refnum<vi>)
            n189 = call "Hide VI Panel.vi"("error in (no error)"=w836, "VI"=w831) -> ("error out"=w835:errorcluster)  [unwired: 9 in]
            n190 = call "Config UI.vi"("error in"=w835) -> ("error out"=w834:errorcluster)  [unwired: 10 in]
            n191 = call "Open VI Panel.vi"("error in (no error)"=w834, "VI"=w831) -> ("error out"=w833:errorcluster)  [unwired: 9 in]
          }
          frame "Update Module ID" {
            # "Update the Current Module ID"
            n192 = Variant To Data(error in=w844, type=T36 {"New ID"=-1} ("Update Module ID Argument"), Variant=w841) -> (data=w839:T36, error out=w843:errorcluster)
            n193 = Unbundle By Name(w839) -> ("New ID"=w837:i32)
            n194 = Bundle By Name(cluster=w842, "Module ID"=w837) -> (w838:T25)
          }
          frame "Tree DQMH Selection" {
            # "search and update DQMH Context Help Indicators"
            n195 = Variant To Data(error in=w866, type=T30 {"Tree Sel"=""} ("Tree DQMH Selection Argument"), Variant=w861) -> (data=w859:T30, error out=w864:errorcluster)
            n196 = Unbundle By Name(w859) -> ("Tree Sel"=w847:string)
            n197 = Unbundle By Name(w858) -> ("Project"=w846:refnum<class "Project.lvclass">)
            n198 = call "Get LVItem by Tag.vi"("error in"=w864, "Tag"=w847, "Project in"=w846) -> ("error out"=w865:errorcluster, "Selected Library"=w848:refnum<class "Library.lvclass">, "Selected VI"=w849:refnum<class "VI.lvclass">)  [unwired: 6 in]
            n199 = property class="Project"(reference=w846) -> ("Accessors:Item Description"=w845:string)  [unwired: 1 in, 2 out]
            n200 = property class="Library"(reference=w848) -> ("Accessors:Item Description"=w853:string, "Accessors:Type"=w852:T26)  [unwired: 1 in, 2 out]
            n201 = property class="VI"(reference=w849) -> (reference out=w856:refnum<class "VI.lvclass">, error out=w862:errorcluster, "Accessors:Item Description"=w851:string)  [unwired: 1 in]
            n202 = Bundle By Name(cluster=w858, "Tree Selection"=w847, "Current Selection.VI"=w849, "Current Selection.Library"=w848) -> (w850:T25)
            n203 = Bundle By Name(cluster=T48 {"Module Description"="", "Event Description"=""} ("Documentation"), "Event Description"=w851, "Module Description"=w853) -> (w855:T48)
            n204 = call "Module Type Updated.vi"("Module Type"=w852) -> ()  [unwired: 10 in, 1 out]
            n205 = call "Get Connector Pane.vi"("error in"=w862, "VI"=w856) -> ("error out"=w863:errorcluster, "Connector Pane"=w857:picture)  [unwired: 8 in]
            n206 = call "Documentation Updated.vi"("Documentation"=w855) -> ()  [unwired: 10 in, 1 out]
            n207 = call "Project Description Updated.vi"("Project Description"=w845) -> ()  [unwired: 10 in, 1 out]
            n208 = call "Connector Pane Updated.vi"("error in"=w863, "Event Connector Pane"=w857) -> ()  [unwired: 9 in, 1 out]
          }
          frame "-------PROJECT----------" {
          }
          frame "Load Project From Path" {
            # "Loads previously scanned project from binary file"
            n209 = Variant To Data(error in=w882, type=T41 {"Project Path"=path ""} ("Load Project From Path Argument"), Variant=w878) -> (data=w876:T41, error out=w880:errorcluster)
            n210 = Unbundle By Name(w876) -> ("Project Path"=w873:path)
            n211 = control-ref of="Modules Tree"() -> (w872:refnum<vi>)
            n212 = call "Load Scan from File Path.vi"("TreeControl in"=w872, "Data Cluster In"=w875, "error in"=w880, "Project Path"=w873) -> ("error out"=w879:errorcluster, "Continue?"=w870:bool, "Data Cluster Out"=w874:T25)  [unwired: 5 in]
            n213 = case shown="False" w870 {
              tunnel: [w885 w887] -> w881
              tunnel: w879 -> [w886 w887]
              tunnel: w871 -> [w884 _]
              frame False {
                n214 = call-poly <vilib>:"Delacor_lib_QMH_Enqueue Message (poly).vi"("error in"=w886, "Message"="Home Screen", "Message Queue in"=w884) -> ("error out"=w885:errorcluster)  [unwired: 7 in, 1 out]
              }
              frame True {
                # "Continue"
              }
            }
            n215 = call "Progress updated.vi"("error in"=w879, "Progress"=i16 -1) -> ()  [unwired: 9 in, 1 out]
          }
          frame "Open Project Folder" {
            n216 = Unbundle By Name(w890) -> ("Project"=w888:refnum<class "Project.lvclass">)
            n217 = property class="Project"(reference=w888) -> ("Accessors:Item Path"=w889:path)  [unwired: 1 in, 2 out]
            n218 = call "Open File on Disk.vi"("error in"=w892, "file or directory path"=w889) -> ("error out"=w891:errorcluster)  [unwired: 9 in]
          }
          frame "Open Project Explorer" {
            # "Open Project Explorer Window"
            n219 = Unbundle By Name(w895) -> ("Project"=w894:refnum<class "Project.lvclass">)
            n220 = property class="Project"(reference=w894, error in=w898) -> (error out=w897:errorcluster, "Accessors:Project Ref"=w893:refnum<vi>)  [unwired: 1 out]
            n221 = invoke class="Project" method="Open Window"(reference=w893, error in=w897) -> (error out=w899:errorcluster)  [unwired: 1 in, 2 out]
            n222 = call "Show Panel.vi"("error in (no error)"=w899) -> ("error out"=w896:errorcluster)  [unwired: 10 in]
          }
          frame "Show Project DQMH Info" {
            n223 = call <vilib>:"Set Busy.vi"("error in (no error)"=w909) -> ()  [unwired: 9 in, 2 out]
            n224 = Unbundle By Name(w905) -> ("Project"=w901:refnum<class "Project.lvclass">)
            n225 = call "Status Updated.vi"("Status"="Parsing Project for DQMH info") -> ()  [unwired: 10 in, 1 out]
            n226 = call "Script Parse Project Modules Constants.vi"("error in"=w909, "Project"=w901) -> ("error out"=w908:errorcluster, "Modules Types"=w900:T26[], "Project info Results"=w902:string[][])  [unwired: 7 in]
            n227 = call "Hide Panel.vi"("error in (no error)"=w908) -> ("error out"=w907:errorcluster)  [unwired: 10 in]
            n228 = call "Insert Module Types.vi"("All Modules types"=w900, "Project info Results In"=w902) -> ("Project info Results Out"=w903:string[][])  [unwired: 9 in]
            n229 = call "Display Project Info Results.vi"("error in"=w907, "Project Results"=w903) -> ("error out"=w906:errorcluster)  [unwired: 9 in]
            n230 = call "Show Panel.vi"("error in (no error)"=w906) -> ("error out"=w910:errorcluster)  [unwired: 10 in]
            n231 = call <vilib>:"Unset Busy.vi"("error in (no error)"=w910) -> ()  [unwired: 10 in, 1 out]
          }
          frame "--------DOCUMENTATION------" {
          }
          frame "Generate Project Documentation" {
            # "#Documentation #Antidoc"
            n232 = Variant To Data(error in=w921, type=T34 {"Boolean"=FALSE} ("Generate Project Documentation Argument"), Variant=w917) -> (error out=w918:errorcluster)  [unwired: 1 out]
            n233 = Unbundle By Name(w915) -> ("Project"=w914:refnum<class "Project.lvclass">)
            n234 = call <vilib>:"Set Busy.vi"("error in (no error)"=w918) -> ()  [unwired: 9 in, 2 out]
            n235 = property class="Project"(reference=w914) -> ("Accessors:Item Path"=w913:path)  [unwired: 1 in, 2 out]
            n236 = call "Generate Documentation--dialog.vi"("error in"=w918, "Project Path"=w913) -> ("error out"=w920:errorcluster)  [unwired: 9 in]
            n237 = Merge Errors(w920) -> (w919:errorcluster)
            n238 = call <vilib>:"Unset Busy.vi"("error in (no error)"=w919) -> ()  [unwired: 10 in, 1 out]
          }
          frame "Save VI Description" {
            # "Save Event Description #Documentation"
            n239 = Variant To Data(error in=w931, type=T38 {"VI Description"=""} ("Save VI Description Argument"), Variant=w927) -> (data=w925:T38, error out=w930:errorcluster)
            n240 = Unbundle By Name(w925) -> ("VI Description"=w923:string)
            n241 = in-place {
              in-place-border: w923 -> [w938]
              in-place-border: [w939] -> w929
              n242 = in-place-cluster #2(w924) -> ("Project"=w934:refnum<class "Project.lvclass">, "Current Selection.Library"=w936:refnum<class "Library.lvclass">, "Current Selection.VI"=w937:refnum<class "VI.lvclass">)
              n243 = call "Save Event Description.vi"("Event Description"=w938, "VI in"=w937) -> ("error out"=w941:errorcluster, "VI Out"=w935:refnum<class "VI.lvclass">)  [unwired: 8 in]
              n244 = call "Update VI in Library.vi"("error in"=w941, "VI"=w935, "Library in"=w936) -> ("error out"=w940:errorcluster, "Library out"=w932:refnum<class "Library.lvclass">)  [unwired: 7 in]
              n245 = call "Update Library.vi"("error in"=w940, "Library"=w932, "Project in"=w934) -> ("error out"=w939:errorcluster, "Project out"=w933:refnum<class "Project.lvclass">)  [unwired: 7 in]
              n246 = in-place-cluster #2("Project"=w933, "Current Selection.Library"=w932, "Current Selection.VI"=w935) -> (w922:T25)
            }
            n247 = Merge Errors(w930, w929) -> (w928:errorcluster)
          }
          frame "Save Library Description" {
            # "Save Library Description #Documentation"
            n248 = Variant To Data(error in=w951, type=T37 {"Library Description"=""} ("Save Library Description Argument"), Variant=w947) -> (data=w945:T37, error out=w950:errorcluster)
            n249 = Unbundle By Name(w945) -> ("Library Description"=w944:string)
            n250 = in-place {
              in-place-border: w944 -> [w956]
              in-place-border: [w957] -> w948
              n251 = in-place-cluster #3(w943) -> ("Project"=w955:refnum<class "Project.lvclass">, "Current Selection.Library"=w953:refnum<class "Library.lvclass">)
              n252 = call "Save Library Documentation.vi"("New Description"=w956, "Library"=w953) -> ("error out"=w957:errorcluster, "Library Out"=w952:refnum<class "Library.lvclass">)  [unwired: 8 in]
              n253 = call "Update Library.vi"("Library"=w952, "Project in"=w955) -> ("Project out"=w954:refnum<class "Project.lvclass">)  [unwired: 8 in, 1 out]
              n254 = in-place-cluster #3("Project"=w954, "Current Selection.Library"=w952) -> (w942:T25)
            }
            n255 = Merge Errors(w950, w948) -> (w949:errorcluster)
          }
          frame "Open Documentation" {
            # "Open #Antidoc #Documentation"
            n256 = Variant To Data(error in=w974, type=T39 {"Boolean"=FALSE} ("Open Documentation Argument"), Variant=w969) -> (error out=w973:errorcluster)  [unwired: 1 out]
            n257 = Unbundle By Name(w962) -> ("Project"=w967:refnum<class "Project.lvclass">)
            n258 = property class="Project"(reference=w967, error in=w973) -> (error out=w972:errorcluster, "Accessors:Item Path"=w961:path)  [unwired: 1 out]
            n259 = call <vilib>:"Get File Extension.vi"("file"=w961) -> ("filename without extension"=w960:string)  [unwired: 6 in, 4 out]
            n260 = Format Into String(format string="Antidoc-Output\\\\%s.pdf", w960) -> (resulting string=w959:string)  [unwired: 2 in, 1 out]
            n261 = Strip Path(path=w961) -> (stripped path=w966:path)  [unwired: 1 out]
            n262 = Build Path(base path=w966, name or relative path=w959) -> (appended path=w965:path)
            n263 = call <vilib>:"Check if File or Folder Exists.vi"("error in (no error)"=w972, "path"=w965) -> ("error out"=w971:errorcluster, "file or folder exists?"=w963:bool, "dup path"=w964:path)  [unwired: 7 in]
            n264 = case shown="False" w963 {
              tunnel: w964 -> [_ w977]
              tunnel: w971 -> [w976 w979]
              tunnel: [w976 w978] -> w970
              frame False {
                # "File not found"
                n265 = invoke on="Generate Antidoc" class="Bool" method="ObjHighlight"() -> ()  [unwired: 3 in, 3 out]
                n266 = call "Status Updated.vi"("Status"="No Antidoc Output found, select a project and Click the Antidoc Icon.") -> ()  [unwired: 10 in, 1 out]
              }
              frame True {
                # "File found, open in default Browser"
                n267 = call-poly <vilib>:"Open URL in Default Browser.vi"("error in (no error)"=w979, "path"=w977) -> ("error out"=w978:errorcluster)  [unwired: 4 in, 1 out]
              }
            }
          }
          frame "Save Project Documentation" {
            # "Save Project description #Documentation"
            n268 = Variant To Data(error in=w988, type=T40 {"Project Description"=""} ("Save Project Documentation Argument"), Variant=w985) -> (data=w983:T40, error out=w987:errorcluster)
            n269 = Unbundle By Name(w983) -> ("Project Description"=w982:string)
            n270 = in-place {
              in-place-border: w987 -> [w997]
              in-place-border: [w994] -> w986
              in-place-border: w982 -> [w991]
              n271 = in-place-cluster #4(w981) -> ("Project"=w989:refnum<class "Project.lvclass">)
              n272 = property class="Project"(reference=w989, error in=w997) -> (reference out=w992:refnum<class "Project.lvclass">, error out=w995:errorcluster, "Accessors:Project Ref"=w993:refnum<vi>)
              n273 = property class="Project"(reference=w993, error in=w995, "Description"=w991) -> (error out=w996:errorcluster)  [unwired: 1 out]
              n274 = property class="Project"(reference=w992, error in=w996, "Accessors:Item Description"=w991) -> (reference out=w990:refnum<class "Project.lvclass">, error out=w994:errorcluster)
              n275 = in-place-cluster #4("Project"=w990) -> (w980:T25)
            }
          }
          frame "---Exit and Error Handling---" {
            # "Separator - The following cases handle errors and exit messages."
          }
          frame "Error" {
            # "Error - Check the error message data and respond accordingly. This message is sent by the \"Error Handler\" VIs at the end of each loop in this application."
            n276 = property on="Property Node" class="Module Admin"(reference=w1001) -> ("Accessors:External Launch"=w1000:bool)  [unwired: 1 in, 2 out]
            n277 = Variant To Data(error in=w1009, type=errorcluster {"status"=FALSE, "code"=0, "source"=""} ("error constant"), Variant=w1003) -> (data=w1010:errorcluster, error out=w1007:errorcluster)
            n278 = call "Error Reported.vi"("Error"=w1010) -> ()  [unwired: 10 in, 1 out]
            n279 = case shown="True" w1000 {
              tunnel: [w1015 _] -> w1006
              tunnel: w1002 -> [w1013 _]
              tunnel: w1010 -> [w1014 _]
              frame False {
                # "If the module is running standalone, then pop up an error dialog and call the \"Exit\" message."
                n280 = call <vilib>:"Simple Error Handler.vi"("error in (no error)"=w1014) -> ()  [unwired: 4 in, 5 out]
                n281 = call-poly <vilib>:"Delacor_lib_QMH_Enqueue Message (poly).vi"("Priority Message? (F)"=TRUE, "Message"="Exit", "Message Queue in"=w1013) -> ("error out"=w1015:errorcluster)  [unwired: 7 in, 1 out]
              }
              frame True {
                # "If the module was launched externally, calling the Error Reported broadcast VI is the only action performed by the \"Error\" message. The module's caller can then process the error appropriately."
              }
            }
            n282 = Merge Errors(w1007, w1006) -> (w1005:errorcluster)
            n283 = local write "error out"(w1005) -> ()
          }
          frame "Exit" {
            w1018 = TRUE  # Write
            w1026 = 91  # 91: not all Exit messages will have an argument
            w1028 = TRUE  # Stop the VI
            # "Release the message queue reference"
            # "Exit - Exit the application."
            n284 = Variant To Data(error in=w1035, type=T33 {"Origin"="", "Exit via Stop Module Req?"=FALSE, "Wait for Module to stop?"=FALSE} ("Stop Argument"), Variant=w1027) -> (data=w1024:T33, error out=w1031:errorcluster)
            n285 = invoke on="Modules Tree" class="Tree (strict)" method="Edit Tree Items.Delete"("Delete Children"=TRUE ("Delete Children?")) -> ()  [unwired: 4 in, 5 out]
            n286 = call <vilib>:"Clear Errors.vi"("error in (no error)"=w1031, "specific error code to clear (0: all)"=w1026) -> ("error out"=w1034:errorcluster)  [unwired: 4 in, 1 out]
            n287 = control-ref of="This VI"() -> (w1023:refnum<vi>)
            n288 = call-dynamic "Delacor_lib_QMH_Release Message Queue.vi"("error in"=w1034, "Message Queue"=w1029) -> ("error out"=w1033:errorcluster)  [unwired: 9 in]
            n289 = call "Handle Exit.vi"("Stop Argument"=w1024, "Admin in"=w1022, "VI reference"=w1023) -> ("error out"=w1030:errorcluster)  [unwired: 7 in, 1 out]
            n290 = Unbundle By Name(w1019) -> ("Project"=w1017:refnum<class "Project.lvclass">)
            n291 = Merge Errors(w1033, w1030) -> (w1032:errorcluster)
            n292 = call "Write Project to File.vi"("Write"=w1018, "Project In"=w1017) -> ("Project Out"=w1016:refnum<class "Project.lvclass">)  [unwired: 7 in, 2 out]
            n293 = call "Error Reported.vi"("Error"=w1032) -> ()  [unwired: 10 in, 1 out]
            n294 = call "Stop Module.vi"("Origin"="Panther Dahsboard Stopped") -> ()  [unwired: 10 in, 1 out]
            n295 = call "Close refs.vi"("Project"=w1016) -> ()  [unwired: 10 in, 1 out]
          }
          frame Default {
            # "'Default' case only runs if there is a message that isn't defined in any of the other cases.  Output a programming error."
            n296 = call "Module Name--constant.vi"() -> ("Module Name"=w1036:string)  [unwired: 11 in]
            n297 = xnode ("Error Ring")("parameter 0"=w1037, "parameter 1"=w1036) -> ("error out"=w1041:errorcluster)
            n298 = Merge Errors(w1039, w1041) -> (w1040:errorcluster)
          }
          frame "Add new Module by Path" {
            # "Adding a Module by path, this is going to be uses by the Scripting hooks"
            n299 = Variant To Data(error in=w1059, type=T44 {"Module Folder"=path "", "Module Name"=""} ("Add new Module by Path Argument"), Variant=w1056) -> (data=w1054:T44, error out=w1058:errorcluster)
            n300 = Unbundle By Name(w1054) -> ("Module Folder"=w1050:path, "Module Name"=w1051:string)
            n301 = in-place {
              in-place-border: w1058 -> [w1066]
              in-place-border: w1051 -> [w1064]
              in-place-border: w1050 -> [w1063]
              in-place-border: [w1065] -> w1057
              n302 = in-place-cluster #5(w1053) -> ("Project"=w1062:refnum<class "Project.lvclass">)
              n303 = control-ref of="Modules Tree"() -> (w1060:refnum<vi>)
              n304 = call "Add Module to Project by Path.vi"("TreeControl in"=w1060, "error in"=w1066, "Module Name"=w1064, "Module Folder"=w1063, "Project"=w1062) -> ("error out"=w1065:errorcluster, "Project Out"=w1061:refnum<class "Project.lvclass">)  [unwired: 5 in]
              n305 = in-place-cluster #5("Project"=w1061) -> (w1052:T25)
            }
          }
          frame "Refresh Module By Name" {
            # "Refresh DQMH Module by Name, this is to be used by the Scripting Hooks"
            n306 = Variant To Data(error in=w1076, type=T45 {"Module Name"=""} ("Refresh Module By Name Argument"), Variant=w1073) -> (data=w1071:T45, error out=w1075:errorcluster)
            n307 = Unbundle By Name(w1071) -> ("Module Name"=w1070:string)
            n308 = control-ref of="Modules Tree"() -> (w1067:refnum<vi>)
            n309 = call "Refresh by Name.vi"("TreeControl in"=w1067, "Data Cluster In"=w1069, "error in"=w1075, "Module Name"=w1070) -> ("error out"=w1074:errorcluster, "Data Cluster Out"=w1068:T25)  [unwired: 6 in]
          }
          frame "Remove Module By Name" {
            # "Remove module by the specified Name, to be used by Scritping Hooks"
            n310 = Variant To Data(error in=w1086, type=T46 {"Module Name"=""} ("Remove Module By Name Argument"), Variant=w1083) -> (data=w1081:T46, error out=w1084:errorcluster)
            n311 = Unbundle By Name(w1081) -> ("Module Name"=w1078:string)
            n312 = control-ref of="Modules Tree"() -> (w1077:refnum<vi>)
            n313 = call "Remove Module from Project by Name.vi"("TreeControl in"=w1077, "error in"=w1084, "Module Name"=w1078, "Data Cluster In"=w1080) -> ("error out"=w1085:errorcluster, "Data Cluster Out"=w1079:T25)  [unwired: 6 in]
          }
        }
        n314 = call-dynamic "Delacor_lib_QMH_Error Handler - Message Handling Loop.vi"("error in"=w465, "Ignore Errors (Runtime)"=w453, "Message Queue in"=w455) -> ("dup error in"=w462:errorcluster)  [unwired: 7 in, 1 out]
      }
      n315 = while {
        tunnel: w29 -> [w99]
        shift-right: [w101] -> w36
        shift-left: w34 -> [w102]
        tunnel: [w103] -> w39
        shift-right: [w98] -> _
        shift-left: w30 -> [w97]
        shift-right: [w96] -> _
        shift-left: Item_Type--enum."» Public API VIs" ("Selection") -> [w95]
        stop <- w100 stop-if-true
        # "Event Handling Loop"
        n316 = event "DQMH_EVENT_MAIN" shown="[0] \"Add Event\", \"Remove Event\", \"Convert Event\", \"Rename Event\", \"Add New Module\", \"Rename Module\", \"Validate Module\", \"Create Module Template\", \"Add Unit Test Module\", \"Create RT Tester Module\", \"Add Helper Loop to Module\", \"Duplicate Event\", \"Duplicate Module\", \"HSE-Ifi Module\": Value Change" {
          selector: w102 -> [_ _ _ _ _ _ _ _ _ _ _ _ _ _ _ _ _ _ _ _ _ _ _ _ _ _ _ _ _ _ _ _ _ _ _ _ _]
          dyn-events: [_ _ _ _ _ _ _ _ _ _ _ _ _ _ _ _ _ _ _ _ _ _ _ _ _ _ _ _ _ _ _ _ _ _ _ _ _] -> w101
          timeout: _ -> [_ _ _ _ _ _ _ _ _ _ _ _ _ _ _ _ _ _ _ _ _ _ _ _ _ _ _ _ _ _ _ _ _ _ _ _ _]
          tunnel: [_ _ _ _ _ _ _ _ _ _ _ _ _ _ TRUE ("Discard?") _ _ _ _ _ _ _ _ _ _ _ _ _ _ _ _ _ _ _ _ _ _] -> w100
          tunnel: w99 -> [w106 _ _ w146 w163 w171 w234 _ w244 _ _ w262 _ _ w286 w295 _ w304 w312 w320 w328 w336 w341 w349 w357 w365 w373 w381 w389 w397 w405 w413 w421 _ w433 w441 w449]
          tunnel: [w112 w137 w142 w147 w164 w172 w235 w240 w245 w249 _ w263 _ w277 w289 w297 _ w307 w315 w323 w331 w339 w344 w352 w360 w368 w376 w384 w392 w400 w408 w416 w424 _ w436 w444 w452] -> w104
          tunnel: [w111 w136 w141 w144 w161 w169 w230 w237 w242 w247 w251 w258 w265 w276 w279 w292 w299 w306 w314 w322 w330 w338 w343 w351 w359 w367 w375 w383 w391 w399 w407 w415 w423 w427 w435 w443 w451] -> w98
          tunnel: w97 -> [w111 w136 w141 w144 w161 w169 _ w237 w242 w247 w251 w258 w265 w276 w279 w292 w299 w306 w314 w322 w330 w338 w343 w351 w359 w367 w375 w383 w391 w399 w407 w415 w423 w427 w435 w443 w451]
          tunnel: [w110 w135 w140 w143 w160 w168 w228 w236 w241 w246 w250 w257 w264 w275 w278 w291 w298 w305 w313 w321 w329 w337 w342 w350 w358 w366 w374 w382 w390 w398 w406 w414 w422 w426 w434 w442 w450] -> w96
          tunnel: w95 -> [w110 w135 w140 _ w160 w168 _ w236 w241 w246 w250 w257 w264 w275 w278 w291 w298 w305 w313 w321 w329 w337 w342 w350 w358 w366 w374 w382 w390 w398 w406 w414 w422 w426 w434 w442 w450]
          event Value Change {
            n317 = event-data() -> ("CtlRef"=w108:refnum<vi>)  [unwired: 1 in]
            n318 = property class="Bool"(reference=w108) -> ("Label.Text"=w109:string)  [unwired: 1 in, 2 out]
            n319 = case shown="\"HSE-Ifi Module\"" w109 {
              tunnel: [DQMH_Tools_Menu--enum."Create New DQMH Event" ("DQMH Tools") _ DQMH_Tools_Menu--enum."Convert DQMH Event" ("DQMH Tools") DQMH_Tools_Menu--enum."Remove DQMH Event" ("DQMH Tools") DQMH_Tools_Menu--enum."Rename DQMH Event" ("DQMH Tools") DQMH_Tools_Menu--enum."Add New DQMH Module" ("DQMH Tools") DQMH_Tools_Menu--enum."Rename DQMH Module" ("DQMH Tools") DQMH_Tools_Menu--enum."HSE-ify DQMH Module" ("DQMH Tools") DQMH_Tools_Menu--enum."Validate DQMH Module" ("DQMH Tools") DQMH_Tools_Menu--enum."Create RT Tester" ("DQMH Tools") DQMH_Tools_Menu--enum."New DQMH  Unit Test" ("DQMH Tools") DQMH_Tools_Menu--enum."Create DQMH Module Template" ("DQMH Tools") DQMH_Tools_Menu--enum."Add Helper Loop to DQMH Module" ("DQMH Tools") DQMH_Tools_Menu--enum."Duplicate Event" ("DQMH Tools") DQMH_Tools_Menu--enum."Duplicate Module" ("DQMH Tools")] -> w107
              tunnel: [_ TRUE _ _ _ _ _ _ _ _ _ _ _ _ _] -> w105
              frame "Add Event" {
              }
              frame Default {
              }
              frame "Convert Event" {
              }
              frame "Remove Event" {
              }
              frame "Rename Event" {
              }
              frame "Add New Module" {
              }
              frame "Rename Module" {
              }
              frame "HSE-Ifi Module" {
              }
              frame "Validate Module" {
              }
              frame "Create RT Tester Module" {
              }
              frame "Add Unit Test Module" {
              }
              frame "Create Module Template" {
              }
              frame "Add Helper Loop to Module" {
              }
              frame "Duplicate Event" {
              }
              frame "Duplicate Module" {
              }
            }
            n320 = case shown="False" w105 {
              tunnel: [w118 _] -> w112
              tunnel: w107 -> [w114 _]
              tunnel: w106 -> [w113 _]
              frame False {
                n321 = Bundle(cluster=T27 {"Scripting Tool"=enum."Create New DQMH Event"} ("Launch DQMH Scripting Tools Argument"), "Scripting Tool"=w114) -> (w117:T27)
                n322 = call-poly <vilib>:"Delacor_lib_QMH_Enqueue Message (poly).vi"("Message Data"=w117, "Message"="Launch DQMH Scripting Tools", "Message Queue in"=w113) -> ("error out"=w118:errorcluster)  [unwired: 7 in, 1 out]
              }
              frame True {
                # "Invalid Label"
              }
            }
          }
          event Value Change {
            # "Open Documentation DQMH Module"
            n323 = event-data() -> ()  [unwired: 1 in, 1 out]
            n324 = case shown="True" "Context Help Panther" {
              tunnel: [w138 w139] -> w137
              frame False {
                n325 = call "Hide Panel.vi"() -> ("error out"=w138:errorcluster)  [unwired: 11 in]
              }
              frame True {
                n326 = call "Show Panel.vi"() -> ("error out"=w139:errorcluster)  [unwired: 11 in]
              }
            }
          }
          event User Event {
            # "We wait for the Context help module to init to send a request to refresh \npanther Dashboard Broadcasts, we need this module to be\nlistening Panther Dashboard broadcasts"
            n327 = event-data() -> ()  [unwired: 1 in, 1 out]
            n328 = call "Refresh Panther Dashboard Broadcasts.vi"() -> ("error out"=w142:errorcluster)  [unwired: 11 in]
          }
          event "Modules Tree": Double Click {
            # "User double click an element on the tree control, we check if it is an event to find its frame on the corresponding DQMH module, we also check if it is a broadcast to find where is being triggered"
            n329 = event-data() -> ("Tag"=w145:string)  [unwired: 1 in]
            n330 = call "Validate if event is selected.vi"("Tree Selection"=w145) -> ("Selection"=w143:T24)  [unwired: 10 in]
            n331 = case shown="\"Requests\"..\"Request and Wait for Reply\"" w143 {
              tunnel: [w150 w153 w156 _ w159] -> w147
              tunnel: w146 -> [w148 w152 w155 _ w158]
              frame "Module" {
                # "Selection is a module"
                n332 = call-poly <vilib>:"Delacor_lib_QMH_Enqueue Message (poly).vi"("Message"="Find Module in project explorer", "Message Queue in"=w148) -> ("error out"=w150:errorcluster)  [unwired: 8 in, 1 out]
              }
              frame "Project" {
                # "Selection is a module"
                n333 = call-poly <vilib>:"Delacor_lib_QMH_Enqueue Message (poly).vi"("Message"="Open Project Explorer", "Message Queue in"=w152) -> ("error out"=w153:errorcluster)  [unwired: 8 in, 1 out]
              }
              frame "Requests".."Request and Wait for Reply" {
                # "Selection is an Event vi?"
                n334 = call-poly <vilib>:"Delacor_lib_QMH_Enqueue Message (poly).vi"("Message"="Locate Event on Main", "Message Queue in"=w155) -> ("error out"=w156:errorcluster)  [unwired: 8 in, 1 out]
              }
              frame Default {
              }
              frame "» Constant VIs", "» Error VIs" {
                # "Selection is either an error or a constant"
                n335 = call-poly <vilib>:"Delacor_lib_QMH_Enqueue Message (poly).vi"("Message"="Open VI BD", "Message Queue in"=w158) -> ("error out"=w159:errorcluster)  [unwired: 8 in, 1 out]
              }
            }
          }
          event "Modules Tree": Drag Starting? {
            # "Drag current selection to user destination"
            n336 = event-data() -> ()  [unwired: 1 in, 1 out]
            n337 = case shown="\"Requests\"..\"Request and Wait for Reply\", \"» Public API VIs\"..\"» Error VIs\"" w160 {
              tunnel: [_ w167] -> w164
              tunnel: w163 -> [_ w166]
              frame Default {
              }
              frame "Requests".."Request and Wait for Reply", "» Public API VIs".."» Error VIs" {
                n338 = call-poly <vilib>:"Delacor_lib_QMH_Enqueue Message (poly).vi"("Message"="Drag VI", "Message Queue in"=w166) -> ("error out"=w167:errorcluster)  [unwired: 8 in, 1 out]
              }
            }
            n339 = event-data("Discard?"=TRUE) -> ()  [unwired: 1 in, 1 out]
          }
          event "Modules Tree": Shortcut Menu Selection (User) {
            # "User selects something from the Right Click Shortcut Menu"
            n340 = event-data() -> ("ItemTag"=w170:string)  [unwired: 1 in]
            n341 = case shown="\"Mod-HSE\"" w170 {
              selector: w170 -> [w175 w181 _ _ _ _ _ _ _ _ _ _ _]
              tunnel: w171 -> [w179 w182 w184 w188 w192 w196 w200 w204 w208 w212 w216 w220 w224]
              tunnel: [w180 w183 w187 w191 w195 w199 w203 w207 w211 w215 w219 w223 w227] -> w172
              frame "-Run: Hide Panel", "-Run: Show Diagram", "-Run: Show Panel", "-Run: Stop Module" {
                n342 = Match Pattern(string=w175, regular expression="-Run: ") -> (after substring=w174:string)  [unwired: 1 in, 3 out]
                n343 = Bundle(cluster=T29 {"Event Name"=""} ("Execute Default Event Request Argument"), "Event Name"=w174) -> (w177:T29)
                n344 = call-poly <vilib>:"Delacor_lib_QMH_Enqueue Message (poly).vi"("Message Data"=w177, "Message"="Execute Default Event Request", "Message Queue in"=w179) -> ("error out"=w180:errorcluster)  [unwired: 7 in, 1 out]
              }
              frame Default {
                n345 = call-poly <vilib>:"Delacor_lib_QMH_Enqueue Message (poly).vi"("Message"=w181, "Message Queue in"=w182) -> ("error out"=w183:errorcluster)  [unwired: 8 in, 1 out]
              }
              frame "Mod-Create Event" {
                n346 = call-poly <vilib>:"Delacor_lib_QMH_Enqueue Message (poly).vi"("Message Data"=T27 {"Scripting Tool"=enum."Create New DQMH Event"} ("Launch DQMH Scripting Tools Argument"), "Message"="Launch DQMH Scripting Tools", "Message Queue in"=w184) -> ("error out"=w187:errorcluster)  [unwired: 7 in, 1 out]
              }
              frame "Mod-Rename" {
                n347 = call-poly <vilib>:"Delacor_lib_QMH_Enqueue Message (poly).vi"("Message Data"=T27 {"Scripting Tool"=enum."Rename DQMH Module"} ("Launch DQMH Scripting Tools Argument"), "Message"="Launch DQMH Scripting Tools", "Message Queue in"=w188) -> ("error out"=w191:errorcluster)  [unwired: 7 in, 1 out]
              }
              frame "Mod-Duplicate" {
                n348 = call-poly <vilib>:"Delacor_lib_QMH_Enqueue Message (poly).vi"("Message Data"=T27 {"Scripting Tool"=enum."Duplicate Module"} ("Launch DQMH Scripting Tools Argument"), "Message"="Launch DQMH Scripting Tools", "Message Queue in"=w192) -> ("error out"=w195:errorcluster)  [unwired: 7 in, 1 out]
              }
              frame "Mod-Validate" {
                n349 = call-poly <vilib>:"Delacor_lib_QMH_Enqueue Message (poly).vi"("Message Data"=T27 {"Scripting Tool"=enum."Validate DQMH Module"} ("Launch DQMH Scripting Tools Argument"), "Message"="Launch DQMH Scripting Tools", "Message Queue in"=w196) -> ("error out"=w199:errorcluster)  [unwired: 7 in, 1 out]
              }
              frame "Add Helper Loop" {
                n350 = call-poly <vilib>:"Delacor_lib_QMH_Enqueue Message (poly).vi"("Message Data"=T27 {"Scripting Tool"=enum."Add Helper Loop to DQMH Module"} ("Launch DQMH Scripting Tools Argument"), "Message"="Launch DQMH Scripting Tools", "Message Queue in"=w200) -> ("error out"=w203:errorcluster)  [unwired: 7 in, 1 out]
              }
              frame "Add New DQMH Module" {
                n351 = call-poly <vilib>:"Delacor_lib_QMH_Enqueue Message (poly).vi"("Message Data"=T27 {"Scripting Tool"=enum."Add New DQMH Module"} ("Launch DQMH Scripting Tools Argument"), "Message"="Launch DQMH Scripting Tools", "Message Queue in"=w204) -> ("error out"=w207:errorcluster)  [unwired: 7 in, 1 out]
              }
              frame "Mod-HSE" {
                n352 = call-poly <vilib>:"Delacor_lib_QMH_Enqueue Message (poly).vi"("Message Data"=T27 {"Scripting Tool"=enum."HSE-ify DQMH Module"} ("Launch DQMH Scripting Tools Argument"), "Message"="Launch DQMH Scripting Tools", "Message Queue in"=w208) -> ("error out"=w211:errorcluster)  [unwired: 7 in, 1 out]
              }
              frame "Rename Event" {
                n353 = call-poly <vilib>:"Delacor_lib_QMH_Enqueue Message (poly).vi"("Message Data"=T27 {"Scripting Tool"=enum."Rename DQMH Event"} ("Launch DQMH Scripting Tools Argument"), "Message"="Launch DQMH Scripting Tools", "Message Queue in"=w212) -> ("error out"=w215:errorcluster)  [unwired: 7 in, 1 out]
              }
              frame "Remove Event" {
                n354 = call-poly <vilib>:"Delacor_lib_QMH_Enqueue Message (poly).vi"("Message Data"=T27 {"Scripting Tool"=enum."Remove DQMH Event"} ("Launch DQMH Scripting Tools Argument"), "Message"="Launch DQMH Scripting Tools", "Message Queue in"=w216) -> ("error out"=w219:errorcluster)  [unwired: 7 in, 1 out]
              }
              frame "Duplicate Event" {
                n355 = call-poly <vilib>:"Delacor_lib_QMH_Enqueue Message (poly).vi"("Message Data"=T27 {"Scripting Tool"=enum."Duplicate Event"} ("Launch DQMH Scripting Tools Argument"), "Message"="Launch DQMH Scripting Tools", "Message Queue in"=w220) -> ("error out"=w223:errorcluster)  [unwired: 7 in, 1 out]
              }
              frame "Convert Event" {
                n356 = call-poly <vilib>:"Delacor_lib_QMH_Enqueue Message (poly).vi"("Message Data"=T27 {"Scripting Tool"=enum."Convert DQMH Event"} ("Launch DQMH Scripting Tools Argument"), "Message"="Launch DQMH Scripting Tools", "Message Queue in"=w224) -> ("error out"=w227:errorcluster)  [unwired: 7 in, 1 out]
              }
            }
          }
          event "Modules Tree": Value Change {
            w230 = TRUE  # Tree valid Selection
            # "The user selected an item on the tree control"
            n357 = event-data() -> ()  [unwired: 1 in, 1 out]
            n358 = Bundle(cluster=T30 {"Tree Sel"=""} ("Tree DQMH Selection Argument"), "Tree Sel"="Modules Tree") -> (w231:T30)
            n359 = call "Validate if event is selected.vi"("Tree Selection"="Modules Tree") -> ("Selection"=w228:T24)  [unwired: 10 in]
            n360 = call-poly <vilib>:"Delacor_lib_QMH_Enqueue Message (poly).vi"("Message Data"=w231, "Message"="Tree DQMH Selection", "Message Queue in"=w234) -> ("error out"=w235:errorcluster)  [unwired: 7 in, 1 out]
          }
          event "Modules Tree": Shortcut Menu Activation? {
            # "This is wher the shorcut menu is filled, only after the user select a module"
            n361 = event-data() -> ("MenuRef"=w239:refnum<k9>)  [unwired: 1 in]
            n362 = call "Create Tree Shortcut Menu.vi"("Selection"=w236, "Menu in"=w239) -> ("error out"=w240:errorcluster)  [unwired: 9 in]
            n363 = Not(x=w237) -> (.not. x?=w238:bool)
            n364 = event-data("Discard?"=w238) -> ()  [unwired: 1 in, 1 out]
          }
          event Value Change {
            # "User wants to go home screen"
            n365 = event-data() -> ()  [unwired: 1 in, 1 out]
            n366 = call-poly <vilib>:"Delacor_lib_QMH_Enqueue Message (poly).vi"("Message"="Home Screen", "Message Queue in"=w244) -> ("error out"=w245:errorcluster)  [unwired: 8 in, 1 out]
          }
          event User Event {
            # "Another Module called the \"Get Module Execution Status\" API Method."
            n367 = event-data() -> ()  [unwired: 1 in, 1 out]
            n368 = call "Update Module Execution Status.vi"("Running?"=TRUE) -> ("error out"=w249:errorcluster)  [unwired: 10 in]
          }
          event User Event {
            # "Hide the panel of this VI, and send a status updated message to let listeners know."
            # "Another Module called the \"Hide Panel\" API Method."
            n369 = event-data() -> ()  [unwired: 1 in, 1 out]
            n370 = control-ref of="This VI"() -> (w252:refnum<vi>)
            n371 = call "Hide VI Panel.vi"("VI"=w252) -> ()  [unwired: 10 in, 1 out]
          }
          event User Event {
            # "Another Module called the \"Scan DQMH Modules\" API Method."
            n372 = event-data() -> ("Include Dependencies"=w256:bool, "Scan All"=w255:bool, "Project"=w254:string, "Target"=w253:string)  [unwired: 1 in]
            n373 = global write "Panther Dashboard--global.vi" "Target"(w253) -> ()
            n374 = Bundle(cluster=T31 {"Include Dependencies"=FALSE, "Scan All"=FALSE, "Project"="", "Target"=""} ("Scan DQMH Modules Argument"), "Include Dependencies"=w256, "Scan All"=w255, "Project"=w254, "Target"=w253) -> (w259:T31)
            n375 = call-poly <vilib>:"Delacor_lib_QMH_Enqueue Message (poly).vi"("Message Data"=w259, "Message"="Scan DQMH Modules", "Message Queue in"=w262) -> ("error out"=w263:errorcluster)  [unwired: 7 in, 1 out]
          }
          event User Event {
            # "Another Module called the \"Show Diagram\" API Method. This event is used for debugging."
            n376 = event-data() -> ()  [unwired: 1 in, 1 out]
            n377 = disable-structure shown="RUN_TIME_ENGINE==False" {
              frame condition #0 (active) {
                # "functionality not available in exe"
                n378 = invoke on="Invoke Node" class="VI" method="Lock State.Get"() -> (error out=w271:errorcluster, "Get Lock State"=w270:T32, "pwd in cache"=w267:bool)  [unwired: 4 in, 1 out]
                n379 = Equal?(x=T32."Password-protected", y=w270) -> (x = y?=w268:bool)
                n380 = Compound Arithmetic op=AND(w268, invert w267) -> (w266:bool)
                n381 = case shown="False" w266 {
                  tunnel: w271 -> [w273 _]
                  frame False {
                    n382 = property on="Property Node" class="VI"(error in=w273, "BDWin.Open"=TRUE ("Block Diagram Window:Open")) -> ()  [unwired: 1 in, 2 out]
                  }
                  frame True {
                    # "Password-protected VI, and the password is not in the cache. Do not show the diagram."
                  }
                }
              }
              frame condition #1 {
              }
            }
          }
          event User Event {
            # "Show the panel of this VI, and send a status updated message to let listeners know."
            # "Another Module called the \"Show Panel\" API Method."
            n383 = event-data() -> ()  [unwired: 1 in, 1 out]
            n384 = control-ref of="This VI"() -> (w274:refnum<vi>)
            n385 = call "Open VI Panel.vi"("VI"=w274) -> ()  [unwired: 10 in, 1 out]
            n386 = call "Register controls Mouse Enter.vi"() -> ("error out"=w277:errorcluster)  [unwired: 11 in]
          }
          event User Event {
            # "The Stop Module Event can get fired from the Exit message in the MHL. The queue gets destroyed in that case. If the queue no longer exists, the Enqueue Exit as a priority message will return error 1. It is safe to ignore, because the module is already exiting."
            # "Another Module called the \"Stop Module\" API Method  or the Message Handling Loop below."
            n387 = event-data() -> ("Exit via Stop Module Req?"=w282:bool, "Wait for Module to stop?"=w281:bool)  [unwired: 1 in]
            n388 = Bundle By Name(cluster=T33 {"Origin"="", "Exit via Stop Module Req?"=FALSE, "Wait for Module to stop?"=FALSE} ("Stop Argument"), "Exit via Stop Module Req?"=w282, "Wait for Module to stop?"=w281) -> (w280:T33)
            n389 = call-poly <vilib>:"Delacor_lib_QMH_Enqueue Message (poly).vi"("Priority Message? (F)"=TRUE, "Message Data"=w280, "Message"="Exit", "Message Queue in"=w286) -> ("error out"=w290:errorcluster)  [unwired: 6 in, 1 out]
            n390 = call <vilib>:"Clear Errors.vi"("error in (no error)"=w290, "specific error code to clear (0: all)"=1) -> ("error out"=w289:errorcluster)  [unwired: 4 in, 1 out]
          }
          event Panel Close? {
            w296 = TRUE  # Discard the event, the MHL is responsible for closing and stopping this VI.
            # "Hide the panel or send the 'Exit' message if the user clicks the 'X' on the module main VI panel."
            n391 = event-data() -> ()  [unwired: 1 in, 1 out]
            n392 = call-poly <vilib>:"Delacor_lib_QMH_Enqueue Message (poly).vi"("Priority Message? (F)"=TRUE, "Message"="Exit", "Message Queue in"=w295) -> ("error out"=w297:errorcluster)  [unwired: 7 in, 1 out]
            n393 = event-data ("Event Filter Node")("Discard?"=w296) -> ()  [unwired: 1 in, 1 out]
          }
          event Timeout {
            n394 = event-data() -> ()  [unwired: 1 in, 1 out]
          }
          event User Event {
            # "Another Module called the \"Launch DQMH Scripting Tools\" API Method."
            n395 = event-data() -> ("Scripting Tool"=w300:T28)  [unwired: 1 in]
            n396 = Bundle(cluster=T27 {"Scripting Tool"=enum."Create New DQMH Event"} ("Launch DQMH Scripting Tools Argument"), "Scripting Tool"=w300) -> (w301:T27)
            n397 = call-poly <vilib>:"Delacor_lib_QMH_Enqueue Message (poly).vi"("Message Data"=w301, "Message"="Launch DQMH Scripting Tools", "Message Queue in"=w304) -> ("error out"=w307:errorcluster)  [unwired: 7 in, 1 out]
          }
          event User Event {
            # "Another Module called the \"Generate Project Documentation\" API Method."
            n398 = event-data() -> ("Boolean"=w308:bool)  [unwired: 1 in]
            n399 = Bundle(cluster=T34 {"Boolean"=FALSE} ("Generate Project Documentation Argument"), "Boolean"=w308) -> (w309:T34)
            n400 = call-poly <vilib>:"Delacor_lib_QMH_Enqueue Message (poly).vi"("Message Data"=w309, "Message"="Generate Project Documentation", "Message Queue in"=w312) -> ("error out"=w315:errorcluster)  [unwired: 7 in, 1 out]
          }
          event Value Change {
            # "Another Module called the \"Generate Project Documentation\" API Method."
            n401 = event-data() -> ()  [unwired: 1 in, 1 out]
            n402 = Bundle(cluster=T34 {"Boolean"=FALSE} ("Generate Project Documentation Argument"), "Boolean"="Generate Antidoc") -> (w317:T34)
            n403 = call-poly <vilib>:"Delacor_lib_QMH_Enqueue Message (poly).vi"("Message Data"=w317, "Message"="Generate Project Documentation", "Message Queue in"=w320) -> ("error out"=w323:errorcluster)  [unwired: 7 in, 1 out]
          }
          event User Event {
            # "Another Module called the \"Show About\" API Method."
            n404 = event-data() -> ("Boolean"=w324:bool)  [unwired: 1 in]
            n405 = Bundle(cluster=T35 {"Boolean"=FALSE} ("Show About Argument"), "Boolean"=w324) -> (w325:T35)
            n406 = call-poly <vilib>:"Delacor_lib_QMH_Enqueue Message (poly).vi"("Message Data"=w325, "Message"="Show About", "Message Queue in"=w328) -> ("error out"=w331:errorcluster)  [unwired: 7 in, 1 out]
          }
          event Value Change {
            # "Another Module called the \"Show About\" API Method."
            n407 = event-data() -> ()  [unwired: 1 in, 1 out]
            n408 = Bundle(cluster=T35 {"Boolean"=FALSE} ("Show About Argument"), "Boolean"="About Panther") -> (w333:T35)
            n409 = call-poly <vilib>:"Delacor_lib_QMH_Enqueue Message (poly).vi"("Message Data"=w333, "Message"="Show About", "Message Queue in"=w336) -> ("error out"=w339:errorcluster)  [unwired: 7 in, 1 out]
          }
          event Value Change {
            # "Another Module called the \"Show About\" API Method."
            n410 = event-data() -> ()  [unwired: 1 in, 2 out]
            n411 = call-poly <vilib>:"Delacor_lib_QMH_Enqueue Message (poly).vi"("Message"="Config UI", "Message Queue in"=w341) -> ("error out"=w344:errorcluster)  [unwired: 8 in, 1 out]
          }
          event User Event {
            # "Another Module called the \"Update Module ID\" API Method."
            n412 = event-data() -> ("New ID"=w345:i32)  [unwired: 1 in]
            n413 = Bundle(cluster=T36 {"New ID"=-1} ("Update Module ID Argument"), "New ID"=w345) -> (w346:T36)
            n414 = call-poly <vilib>:"Delacor_lib_QMH_Enqueue Message (poly).vi"("Message Data"=w346, "Message"="Update Module ID", "Message Queue in"=w349) -> ("error out"=w352:errorcluster)  [unwired: 7 in, 1 out]
          }
          event "Module ID": Value Change {
            # "Another Module called the \"Update Module ID\" API Method."
            n415 = event-data() -> ()  [unwired: 1 in, 1 out]
            n416 = Bundle(cluster=T36 {"New ID"=-1} ("Update Module ID Argument"), "New ID"="Module ID") -> (w354:T36)
            n417 = call-poly <vilib>:"Delacor_lib_QMH_Enqueue Message (poly).vi"("Message Data"=w354, "Message"="Update Module ID", "Message Queue in"=w357) -> ("error out"=w360:errorcluster)  [unwired: 7 in, 1 out]
          }
          event User Event {
            # "Another Module called the \"Save Library Description\" API Method."
            n418 = event-data() -> ("Library Description"=w361:string)  [unwired: 1 in]
            n419 = Bundle(cluster=T37 {"Library Description"=""} ("Save Library Description Argument"), "Library Description"=w361) -> (w362:T37)
            n420 = call-poly <vilib>:"Delacor_lib_QMH_Enqueue Message (poly).vi"("Message Data"=w362, "Message"="Save Library Description", "Message Queue in"=w365) -> ("error out"=w368:errorcluster)  [unwired: 7 in, 1 out]
          }
          event User Event {
            # "Another Module called the \"Save VI Description\" API Method."
            n421 = event-data() -> ("VI Description"=w369:string)  [unwired: 1 in]
            n422 = Bundle(cluster=T38 {"VI Description"=""} ("Save VI Description Argument"), "VI Description"=w369) -> (w370:T38)
            n423 = call-poly <vilib>:"Delacor_lib_QMH_Enqueue Message (poly).vi"("Message Data"=w370, "Message"="Save VI Description", "Message Queue in"=w373) -> ("error out"=w376:errorcluster)  [unwired: 7 in, 1 out]
          }
          event User Event {
            # "Another Module called the \"Open Documentation\" API Method."
            n424 = event-data() -> ("Boolean"=w377:bool)  [unwired: 1 in]
            n425 = Bundle(cluster=T39 {"Boolean"=FALSE} ("Open Documentation Argument"), "Boolean"=w377) -> (w378:T39)
            n426 = call-poly <vilib>:"Delacor_lib_QMH_Enqueue Message (poly).vi"("Message Data"=w378, "Message"="Open Documentation", "Message Queue in"=w381) -> ("error out"=w384:errorcluster)  [unwired: 7 in, 1 out]
          }
          event Value Change {
            # "Another Module called the \"Open Documentation\" API Method."
            n427 = event-data() -> ()  [unwired: 1 in, 1 out]
            n428 = Bundle(cluster=T39 {"Boolean"=FALSE} ("Open Documentation Argument"), "Boolean"="Open Antidoc Output") -> (w386:T39)
            n429 = call-poly <vilib>:"Delacor_lib_QMH_Enqueue Message (poly).vi"("Message Data"=w386, "Message"="Open Documentation", "Message Queue in"=w389) -> ("error out"=w392:errorcluster)  [unwired: 7 in, 1 out]
          }
          event User Event {
            # "Another Module called the \"Save Project Documentation\" API Method."
            n430 = event-data() -> ("Project Description"=w393:string)  [unwired: 1 in]
            n431 = Bundle(cluster=T40 {"Project Description"=""} ("Save Project Documentation Argument"), "Project Description"=w393) -> (w394:T40)
            n432 = call-poly <vilib>:"Delacor_lib_QMH_Enqueue Message (poly).vi"("Message Data"=w394, "Message"="Save Project Documentation", "Message Queue in"=w397) -> ("error out"=w400:errorcluster)  [unwired: 7 in, 1 out]
          }
          event User Event {
            # "Another Module called the \"Load Project From Path\" API Method."
            n433 = event-data() -> ("Project Path"=w401:path)  [unwired: 1 in]
            n434 = Bundle(cluster=T41 {"Project Path"=path ""} ("Load Project From Path Argument"), "Project Path"=w401) -> (w402:T41)
            n435 = call-poly <vilib>:"Delacor_lib_QMH_Enqueue Message (poly).vi"("Message Data"=w402, "Message"="Load Project From Path", "Message Queue in"=w405) -> ("error out"=w408:errorcluster)  [unwired: 7 in, 1 out]
          }
          event User Event {
            # "Another Module called the \"Add DQMH Module to Current Scan\" API Method."
            n436 = event-data() -> ("Include Dependencies"=w409:bool)  [unwired: 1 in]
            n437 = Bundle(cluster=T42 {"Include Dependencies"=FALSE} ("Add DQMH Module to Current Scan Argument"), "Include Dependencies"=w409) -> (w410:T42)
            n438 = call-poly <vilib>:"Delacor_lib_QMH_Enqueue Message (poly).vi"("Message Data"=w410, "Message"="Add DQMH Module to Current Scan", "Message Queue in"=w413) -> ("error out"=w416:errorcluster)  [unwired: 7 in, 1 out]
          }
          event User Event {
            # "Another Module called the \"Highlight Item\" API Method."
            n439 = event-data() -> ("Item Tag"=w417:string)  [unwired: 1 in]
            n440 = Bundle(cluster=T43 {"Item Tag"=""} ("Highlight Item Argument"), "Item Tag"=w417) -> (w418:T43)
            n441 = call-poly <vilib>:"Delacor_lib_QMH_Enqueue Message (poly).vi"("Message Data"=w418, "Message"="Highlight Item", "Message Queue in"=w421) -> ("error out"=w424:errorcluster)  [unwired: 7 in, 1 out]
          }
          event User Event {
            # "Another Module called the \"Update Status\" API Method."
            n442 = event-data() -> ("Status"=w425:string)  [unwired: 1 in]
            n443 = call "Status Updated.vi"("Status"=w425) -> ()  [unwired: 10 in, 1 out]
          }
          event User Event {
            # "Another Module called the \"Add new Module by Path\" API Method."
            n444 = event-data() -> ("Module Folder"=w429:path, "Module Name"=w428:string)  [unwired: 1 in]
            n445 = Bundle(cluster=T44 {"Module Folder"=path "", "Module Name"=""} ("Add new Module by Path Argument"), "Module Folder"=w429, "Module Name"=w428) -> (w430:T44)
            n446 = call-poly <vilib>:"Delacor_lib_QMH_Enqueue Message (poly).vi"("Message Data"=w430, "Message"="Add new Module by Path", "Message Queue in"=w433) -> ("error out"=w436:errorcluster)  [unwired: 7 in, 1 out]
          }
          event User Event {
            # "Another Module called the \"Refresh Module By Name\" API Method."
            n447 = event-data() -> ("Module Name"=w437:string)  [unwired: 1 in]
            n448 = Bundle(cluster=T45 {"Module Name"=""} ("Refresh Module By Name Argument"), "Module Name"=w437) -> (w438:T45)
            n449 = call-poly <vilib>:"Delacor_lib_QMH_Enqueue Message (poly).vi"("Message Data"=w438, "Message"="Refresh Module By Name", "Message Queue in"=w441) -> ("error out"=w444:errorcluster)  [unwired: 7 in, 1 out]
          }
          event User Event {
            # "Another Module called the \"Remove Module By Name\" API Method."
            n450 = event-data() -> ("Module Name"=w445:string)  [unwired: 1 in]
            n451 = Bundle(cluster=T46 {"Module Name"=""} ("Remove Module By Name Argument"), "Module Name"=w445) -> (w446:T46)
            n452 = call-poly <vilib>:"Delacor_lib_QMH_Enqueue Message (poly).vi"("Message Data"=w446, "Message"="Remove Module By Name", "Message Queue in"=w449) -> ("error out"=w452:errorcluster)  [unwired: 7 in, 1 out]
          }
        }
        n453 = call-dynamic "Delacor_lib_QMH_Error Handler - Event Handling Loop.vi"("error in"=w104, "Message Queue in"=w99) -> ("dup error in"=w103:errorcluster)  [unwired: 8 in, 1 out]
      }
      n454 = while {
        tunnel: w33 -> [w51]
        tunnel: [w50] -> w32
        shift-right: [w48] -> _
        shift-left: -1 -> [w47]
        tunnel: w29 -> [w46]
        tunnel: [w52] -> w37
        shift-right: [w45] -> _
        shift-left: _ -> [w44]
        tunnel: w29 -> [w43]
        tunnel: w28 -> [w41]
        stop <- w49 stop-if-true
        # "PDash Modules Monitoring Loop"
        n455 = event shown="[0] Timeout" {
          selector: w51 -> [_ _ _ _ _ w80 _ _ _]
          dyn-events: [_ _ _ _ _ w79 _ _ _] -> w50
          timeout: w47 -> [_ _ _ _ _ _ _ _ _]
          tunnel: [_ TRUE _ _ _ _ _ _ _] -> w49
          tunnel: [w55 w59 w62 w68 w73 w81 w85 w91 w94] -> w48
          tunnel: w47 -> [w55 w59 _ w68 w73 w81 w85 w91 w94]
          tunnel: [w56 _ _ _ _ _ w86 _ _] -> w53
          tunnel: [w54 w58 w64 w67 w69 w75 w82 w89 w93] -> w45
          tunnel: w44 -> [w54 w58 _ w67 w69 w75 w82 w89 w93]
          tunnel: w43 -> [_ _ _ _ _ _ _ _ _]
          tunnel: w41 -> [_ _ _ _ _ _ _ _ _]
          event Timeout {
            n456 = event-data() -> ()  [unwired: 1 in, 1 out]
            n457 = call "Get Module Execution Status by ref.vi"("Helper Loop Cluster"=w54) -> ("error out"=w56:errorcluster)  [unwired: 10 in]
          }
          event User Event {
            n458 = event-data() -> ()  [unwired: 1 in, 1 out]
            n459 = Unbundle By Name(w58) -> ("Main.vi Refs"=w57:refnum<vi>[])
            n460 = Close Reference(reference=w57) -> ()  [unwired: 1 in, 1 out]
          }
          event User Event {
            n461 = event-data() -> ("Project"=w63:refnum<class "Project.lvclass">)  [unwired: 1 in]
            n462 = control-ref of="Modules Tree"() -> (w61:refnum<vi>)
            n463 = call "Get Main VI Refs.vi"("TreeControl in"=w61, "Project"=w63) -> ("HL Cluster"=w64:T51, "Refresh Time"=w62:i32)  [unwired: 7 in, 1 out]
          }
          event User Event {
            n464 = event-data() -> ("Progress"=w66:i16)  [unwired: 1 in]
            "Progress" <- w66
            n465 = Greater Or Equal To 0?(x=w66) -> (x >= 0?=w65:bool)
            n466 = property on="Progress" class="Slide (strict)"("Visible"=w65) -> ()  [unwired: 2 in, 2 out]
          }
          event Mouse Enter {
            n467 = event-data() -> ("CtlRef"=w70:refnum<vi>)  [unwired: 1 in]
            n468 = property class="Ctl"(reference=w70) -> ("TipStrip"=w71:string)  [unwired: 1 in, 2 out]
            n469 = Empty String/Path?(string/path=w71) -> (empty?=w72:bool)
            n470 = case shown="True" w72 {
              tunnel: w71 -> [w74 _]
              frame False {
                n471 = call "Status Updated.vi"("Status"=w74) -> ()  [unwired: 10 in, 1 out]
              }
              frame True {
              }
            }
          }
          event User Event {
            n472 = event-data() -> ()  [unwired: 1 in, 1 out]
            n473 = control-ref of="This VI"() -> (w77:refnum<vi>)
            n474 = property class="VI"(reference=w77) -> ("Panel"=w78:refnum<vi>)  [unwired: 1 in, 2 out]
            n475 = property class="Pnl"(reference=w78) -> ("Controls[]"=w76:refnum<vi>[])  [unwired: 1 in, 2 out]
            n476 = register-events(reference=w80, w76) -> (reference out=w79:refnum<event-registration>)  [unwired: 3 in, 1 out]
          }
          event User Event {
            n477 = event-data() -> ("Scale Max"=w84:i32)  [unwired: 1 in]
            n478 = control-ref of="Progress"() -> (w83:refnum<vi>)
            n479 = property class="Slide (strict)"(reference=w83, "Scale.Maximum"=w84) -> (error out=w86:errorcluster)  [unwired: 1 in, 1 out]
          }
          event User Event {
            n480 = event-data() -> ("Module Type"=w88:T26)  [unwired: 1 in]
            n481 = Equal?(x=Module_type--enum."Cloneable", y=w88) -> (x = y?=w87:bool)
            n482 = property on="Module ID" class="DigNum (strict)"("Visible"=w87) -> ()  [unwired: 2 in, 2 out]
          }
          event User Event {
            n483 = event-data() -> ("Status"=→"String Control":string)  [unwired: 1 in]
          }
        }
        n484 = call-dynamic "Delacor_lib_QMH_Error Handler - Helper Loop.vi"("Error Debug"="PDash Modules Monitoring Loop" ("DQMH_HELPER_LOOP_NAME"), "error in"=w53, "Message Queue in"=w46) -> ("dup error in"=w52:errorcluster)  [unwired: 7 in, 1 out]
      }
    }
    frame Error {
      # "Synchronize Caller Events.vi will inform Start Module.vi that the module has launched and will let the code calling Start Module.vi register for broadcasts and would permit the caller receive the broadcast that an error occurred at launch time."
      n485 = call-dynamic "Delacor_lib_QMH_Release Message Queue.vi"("error in"=w1095, "Message Queue"=w1089) -> ("error out"=w1094:errorcluster)  [unwired: 9 in]
      n486 = call "Synchronize Caller Events.vi"("Singleton Module Admin in"=w1090) -> ("error out"=w1096:errorcluster)  [unwired: 9 in, 1 out]
      n487 = call "Module Name--constant.vi"() -> ("Module Name"=w1092:string)  [unwired: 11 in]
      n488 = Format Into String(format string="An error occurred during initialization. %s is no longer running.", w1092) -> (resulting string=w1087:string)  [unwired: 2 in, 1 out]
      n489 = Merge Errors(w1094, w1096) -> (w1097:errorcluster)
      n490 = call "Stop Module.vi"("Origin"=w1087) -> ()  [unwired: 10 in, 1 out]
      n491 = call "Error Reported.vi"("Additional Information"=w1087, "Error"=w1097) -> ()  [unwired: 9 in, 1 out]
    }
  }
  n492 = Merge Errors(w24, w26, w19) -> (w23:errorcluster)
  n493 = call "Close Module.vi"("error in (no error)"=w23, "Module Admin in"=w14) -> ("error out"=w25:errorcluster, "External Launch"=w8:bool, "Module Admin out"=w9:refnum<class "Delacor_lib_QMH_Module Admin.lvclass">)  [unwired: 7 in]
  n494 = Unregister For Events(event registration refnum=w6) -> ()  [unwired: 1 in, 1 out]
  n495 = Unregister For Events(event registration refnum=w13, error in=w25) -> (error out=w22:errorcluster)
  "error out" <- w22
  n496 = case "External Launch?" shown="True" w8 {
    tunnel: w22 -> [_ w1098]
    frame False {
    }
    frame True {
      n497 = case shown="Error" w1098 {
        frame No Error {
          n498 = invoke class="VI" method="FP.Close"() -> ()  [unwired: 3 in, 3 out]
        }
        frame Error {
          n499 = disable-structure shown="Default" {
            frame condition #0 (active) {
              n500 = invoke class="VI" method="FP.Open"("Activate"=TRUE ("Activate?")) -> ()  [unwired: 4 in, 5 out]
            }
            frame condition #1 {
              # "Don't show panel on error if running inside a built EXE."
            }
          }
        }
      }
    }
  }
  n501 = local write "Module Admin"(w9) -> ()
